vi "plcHMI_rev3.vi"() -> ()   [LabVIEW 2020]
doc: "ADS continuos synchronous write example using base blocks. \n\nThe client writes data synchronously and does wait for the respose from server."
uses:
  Agilent/AgilentTotalCluster.ctl
  Agilent/AgilentControl.ctl
  Agilent/Channel Config.ctl
  <vilib>/Platform/TimedLoop/XDataNode/timing_clust.ctl
  <vilib>/Platform/TimedLoop/XDataNode/nitl_modes.ctl
  <vilib>/Platform/TimedLoop/XDataNode/wakeup.ctl
  <userlib>/Beckhoff-LabVIEW-Interface/_DependsOn/With TypeResolving/Write Sync Single TypeResolved.vi
  <userlib>/Beckhoff-LabVIEW-Interface/_DependsOn/With TypeResolving/Read Sync Single TypeResolved.vi
  <vilib>/Platform/TimedLoop/XDataNode/XDataNode.xnode
  <vilib>/Platform/TimedLoop/XDataNode/XDNodeRunTimeDep.lvlib
panel:
  in  "Tab Control":T1(tab)
  out "error out":errorcluster
  in  "Symbol file path - MUST BE ENTERED\nLoad \"ADS Write AND Read Symbols REV X.X.xml\"":path
  out "bHasMached":bool
  out "Write Status":bool
  out "Read Status":bool
  in  "EXIT HMI":bool caption="STOP HMI\nEXIT HMI"
  out "Internal TwinCAT Handle ID Maps":dbl format="%#_12g"
  in  "802L TDK PSU Voltage Rating (abs(Volts))":i32=12000 min=1 max=50000
  in  "802L TDL PSU Peak Power (J/s)":i32=9000 min=1 max=50000
  in  "HVPS Model":u16(ring) items=["802L-12kV,9000J/s", "802L+50kV,9000J/s", "Other"]
  out "Test Interval Fault":bool
  in  "Cycle Time (Sec)":i32=15 min=0
  in  "Voltage Held by PSU":bool
  in  "Log Capacitor Voltage":bool
  in  "Log Temperature Data":bool
  out "Time Since Last Shot":string caption="Elapsed Time Text"
  in  "Duty Cycle":dbl
  in  "Current Control":bool
  out "Expected Voltage":i16
  in  "Dump":bool
  out "EOC":bool
  out "Maximum Test Number Reached":bool
  out "SCR Ready":bool
  in  "START":bool
  in  "STOP":bool
  in  "Hold":bool
  in  "Charge":bool
  in  "Shot":bool
  in  "HV Switch Mode":bool
  in  "CLEAR FAULT":bool
  in  "Manual/Auto":bool=TRUE
  out "Test Interval (Sec)":i32=15 min=0
  in  "Capacitance (uF)":sgl=1e-13 min=0 max=10000 format="%#_6f"
  in  "Target Charge Volt (V) - Min 1500V - TEMPORARY LIMIT 12kV":i32 min=-12000 max=12000 step=1
  out "Estimated Charge Time (seconds)":sgl
  in  "Hold Time Before Shot (seconds)":sgl max=1000
  in  "Max Number of Shots (Test intervals)":i16=1 min=1
  out "Shot Number":i16
  out "Charge Fault":bool=TRUE
  out "Discharge Fault":bool=TRUE
  out "Hold Fault":bool=TRUE
  out "Cap 1 Temp\nExceeded Fault":bool=TRUE
  out "Ambient Temp\nExceeded Fault":bool=TRUE
  out "PSU Fault":bool=TRUE
  out "Control Sys Fault":bool=TRUE
  out "test Running":bool
  out "Test State":string
  out "Cap 1 Voltage":i16
  out "Cap 1 Temperature":i16
  in  "Capacitor Voltage Data Log File Path (.xlsx)":path
  out "Load Temperature":i16
  out "Soft Dump Temp":i16
  out "Ambient Temp":i16
  out "Waveform Chart - Capacitor Voltage (Probe, abs(Volts))":dbl(graph)
  in  "Manual Charge Time (seconds)":sgl max=90
  in  "Reset Test Number":bool
  in  "Cap 1 Fault Temp (Cel)":i16 min=0 max=125
  in  "Capacitor Temperature Data Log File Path (.xlsx)":path
  out "Cap 1 Voltage (HVPS)":i16
  out "Capacitor Voltage":cluster{dbl, dbl}(graph)
  out "EOC":i16(graph)
  out "Soft Exception":bool
  out "PSU HV FB Fault":bool
  out "Charge FB Fault":bool
  out "Softdump FB Fault":bool
  out "SCR FB":i16(graph)
  in  "CH4 Vertical Units":string(combo)="V"
  in  "CH4 Vertical Units/div":dbl=2.0
  in  "Toggle Scope Scale":bool
  in  "CH1 Vertical Units/div":dbl=2.0
  in  "CH1 Vertical Units":string(combo)="V"
  in  "Horizontal Units":enum16{"us", "ms", "s"}(ring)
  in  "Horizontal Units/div":dbl=200.0
  out "Download":bool
  in  "Single":bool
  in  "Stop":bool
  out "Scope Trig":bool
  in  "Agilent Array":T2[](array[typedef])
  out "Process Step":u8
  in  "C:\\HVTest\\Local_Cap_Log_Scope (.xlsx)":path
  out "Stop Loops":bool
  # "CONFIGURATION"
  # "Press STOP HMI instead of\nLabView Abort Execution"
  # "PSU V Rating, Peak Power\nactive when OTHER\nis selected"
  # "INPUT VARIABLES - For TDK Lambda 802L\nMust be written to before START"
  # "FAULT STATUSES"
  # "Set to -1 for automated\nfull charge to setpoint"
  # "MANUAL CONTROLS"
  # "Does not record during \"wait\" and appends to data file. Must be named with .xlsx"
  # "HV Switch Configuration"
  # "Records during \"Test Running.\" Must be named with .xlsx"
  # "Control Sys Faults"
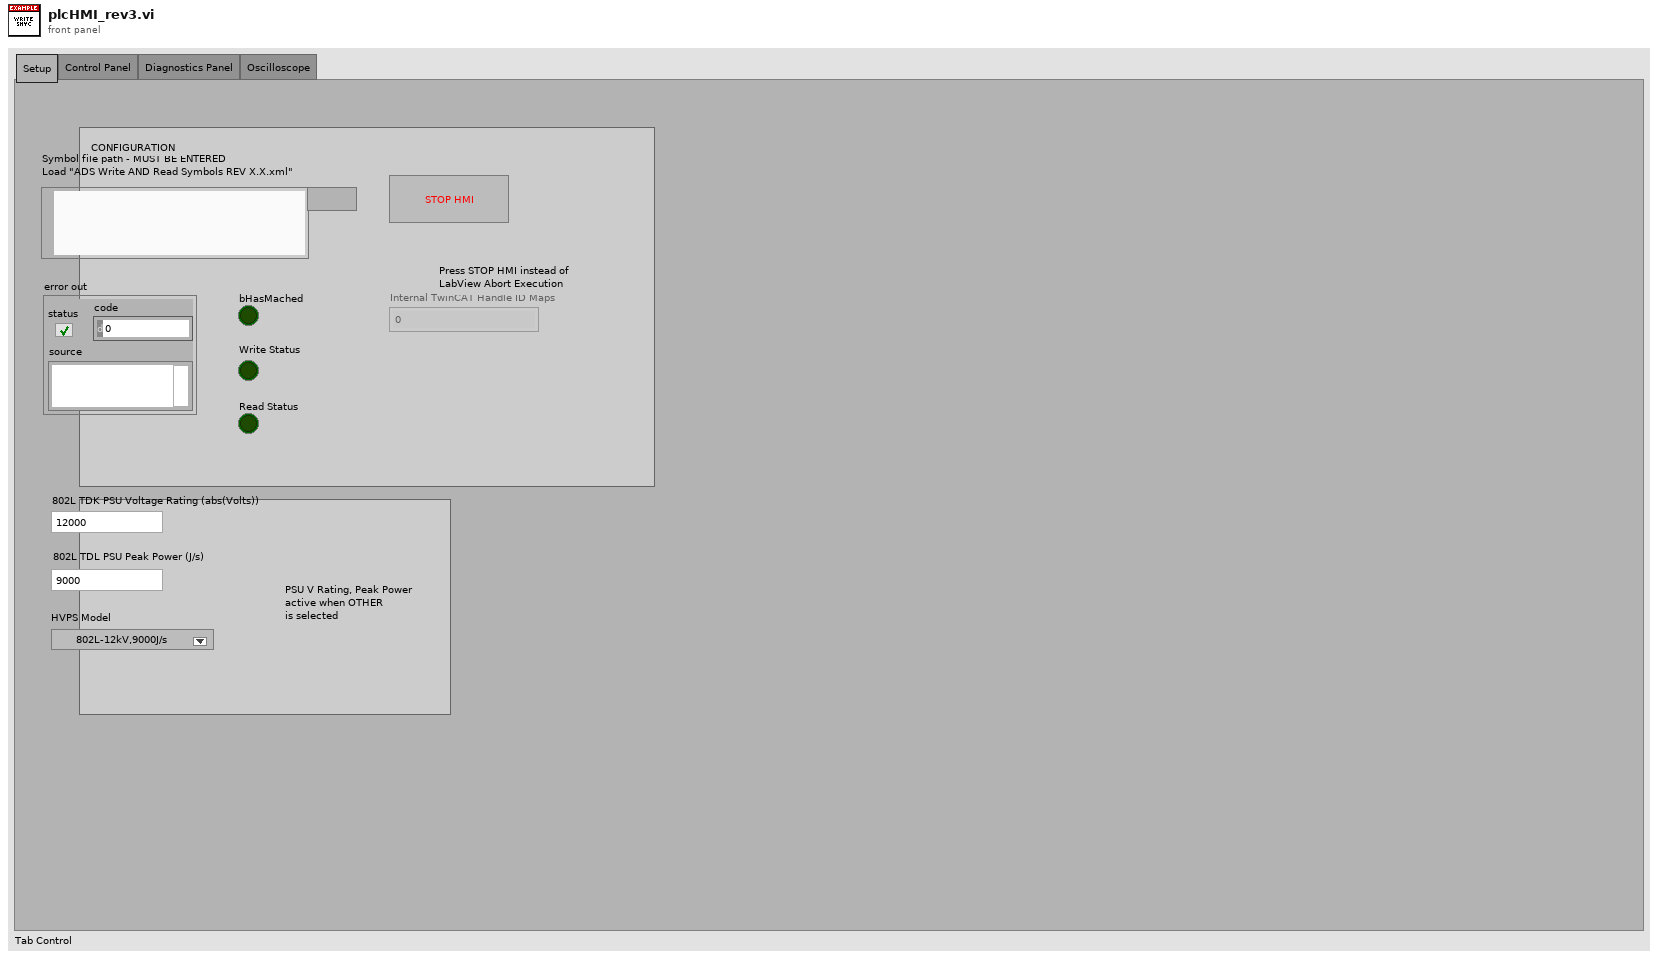
[diagram p1: front panel]
types:
  T1 = enum32{"Setup", "Control Panel", "Diagnostics Panel", "Oscilloscope"}
  T2 = typedef "AgilentTotalCluster.ctl" = cluster{"Agilent Graph":waveform(dbl)[], "Agilent Control":T3, "Agilent Setup Error":errorcluster, "Agilent Present":bool, "Enabled":bool}
  T3 = typedef "AgilentControl.ctl" = cluster{"Trig?":bool, "VISA session":refnum<visa-resource-name>, "Setup to Load":string, "Timeout (ms)":u32, "Desired Samp":enum32{"100", "250", "500", "1000", "2000", "5000", "10000", "20000", "50000", "100000", "200000", "500000", "1000000", "2000000", "4000000", "8000000"}, "Captured Samp":i32, "Desired Channels":T4[]}
  T4 = typedef "Channel Config.ctl" = cluster{"Chan Index":enum16{"Channel1", "Channel2", "Channel3", "Channel4", "MATH"}, "Name":string, "Samples":i32}
  T5 = typedef "XDNodeRunTimeDep.lvlib/timing_clust.ctl" = cluster{"Expected End [f-1]":u64, "Actual End [f-1]":u64, "Finished Late? [f-1]":bool, "Expected End [i-1]":u64, "Actual End [i-1]":u64, "Finished Late? [i-1]":bool, "Expected Start [i]":u64, "Actual Start [i]":u64, "Expected Start [f]":u64, "Actual Start [f]":u64, "Source Name":string, "Structure Name":string, "Period":i64, "Deadline":i64, "Offset":i64, "Start":i64, "Priority":i32, "Timeout":i32, "Mode":T6, "Wakeup Reason":T7, "Error":errorcluster, "Source Type":string, "Secondary Source Type":string, "Global End Time":u64, "Global Start Time":u64, "Frame Duration":u64, "Iteration Duration":u64, "Assigned CPU":i32, "I/O Scan Engine Mode":u32}
  T6 = typedef "XDNodeRunTimeDep.lvlib/nitl_modes.ctl" = enum32{"No Change", "Process missed periods, maintain original phase", "Discard missed periods, maintain original phase", "Process missed periods, ignore original phase", "Discard missed periods, ignore original phase"}
  T7 = typedef "XDNodeRunTimeDep.lvlib/wakeup.ctl" = enum32{"Normal", "Aborted", "Asynchronous wakeup", "Timing source error", "Timed loop error", "Timeout"}
  T8 = cluster{"Agilent Array[0]":T2, "Agilent Array[1]":T2, "Agilent Array[2]":T2, "Agilent Array[3]":T2, "Agilent Array[4]":T2, "Agilent Array[5]":T2, "Agilent Array[6]":T2, "Agilent Array[7]":T2, "Agilent Array[8]":T2}
  T9 = enum32{"100", "250", "500", "1000", "2000", "5000", "10000", "20000", "50000", "100000", "200000", "500000", "1000000", "2000000", "4000000", "8000000"}
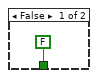
[diagram p2: hidden frame]
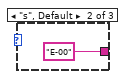
[diagram p5: hidden frame]
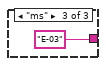
[diagram p6: hidden frame]
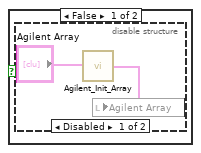
[diagram p7: hidden frame]
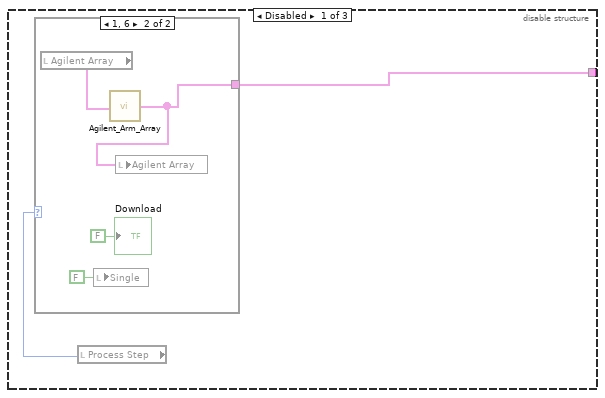
[diagram p11: hidden frame]
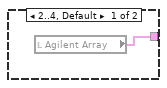
[diagram p12: hidden frame]
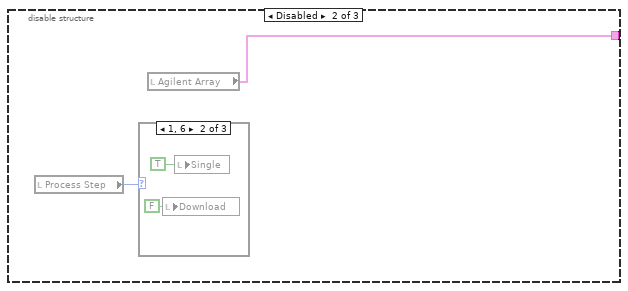
[diagram p13: hidden frame]
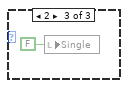
[diagram p15: hidden frame]
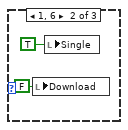
[diagram p17: hidden frame]
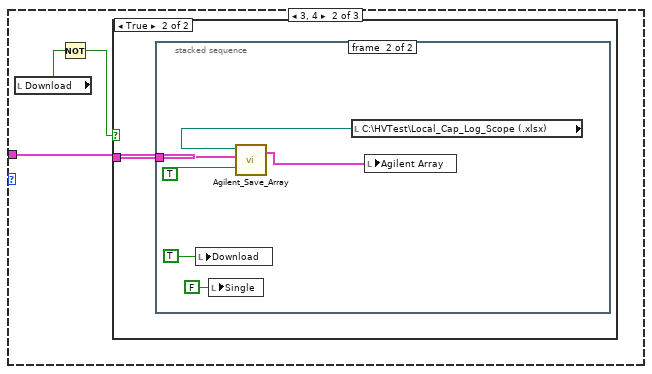
[diagram p19: hidden frame]
diagram:
  w105 = u16 17 items=["SyncLatest"=17, "AsyncLatest"=33] ("WriterMode")
  w189 = u16 33 items=["SyncLatest"=17, "AsyncLatest"=33] ("WriterMode")
  w228 = u16 33 items=["SyncLatest"=17, "AsyncLatest"=33] ("WriterMode")
  w247 = u16 33 items=["SyncLatest"=17, "AsyncLatest"=33] ("WriterMode")
  w266 = u16 33 items=["SyncLatest"=17, "AsyncLatest"=33] ("WriterMode")
  w285 = u16 33 items=["SyncLatest"=17, "AsyncLatest"=33] ("WriterMode")
  w304 = u16 33 items=["SyncLatest"=17, "AsyncLatest"=33] ("WriterMode")
  w323 = u16 33 items=["SyncLatest"=17, "AsyncLatest"=33] ("WriterMode")
  w342 = u16 17 items=["SyncLatest"=17, "AsyncLatest"=33] ("WriterMode")
  w361 = u16 17 items=["SyncLatest"=17, "AsyncLatest"=33] ("WriterMode")
  w380 = u16 17 items=["SyncLatest"=17, "AsyncLatest"=33] ("WriterMode")
  w399 = u16 17 items=["SyncLatest"=17, "AsyncLatest"=33] ("WriterMode")
  w418 = u16 17 items=["SyncLatest"=17, "AsyncLatest"=33] ("WriterMode")
  w437 = u16 17 items=["SyncLatest"=17, "AsyncLatest"=33] ("WriterMode")
  w456 = u16 17 items=["SyncLatest"=17, "AsyncLatest"=33] ("WriterMode")
  w471 = u16 17 items=["SyncLatest"=17, "AsyncLatest"=33] ("WriterMode")
  # "Variables/ Control"
  # "Documentation:\nCode separated vertically into two main sections - Write and read\nThey are further separated into BOOL and numeric\nThe OR gates wire all the error lines and the EXIT HMI button to a WHILE LOOP STOP\nThere current delay time on the routine is 100ms\nAll the AND gates connect the typecast resolve lines to the bHasMatched indicator\nThe second and third set of AND gates connect the write statuses to the Write Status indicator\nThe same is done for the read status indicator"
  # "WRITE NUMERICS"
  # "WRITE BOOLS"
  # "Select Symbol N"
  # "Read Initialization"
  # "Release \nTypeResolver"
  # "Release Writer"
  # "Send Request"
  # "Init \nTypeResolver"
  # "Init Writer"
  # "Select Symbol"
  # "Initialization"
  # "Call Release handle block\nat the end, when all nodes\nhave finished their execution"
  # "There must be only one release\nafter every init block.\nRelease block must be called\nalways at the end."
  # "Release"
  # "Symbol Interface"
  n1 = disable-structure shown="Enabled" {
    disable-tunnel: [w477 _] -> w475
    disable-tunnel: [w476 w479] -> w474
    frame Disabled {
      # "Using Symbol Interface"
      n2 = call <userlib>:"Symbol Interface.vi"() -> ("PortInfo"=w476:string, "error out"=w477:errorcluster)  [unwired: 14 in]
    }
    frame Enabled {
      # "Using Symbol File"
      n3 = Path To String(path="Symbol file path - MUST BE ENTERED\nLoad \"ADS Write AND Read Symbols REV X.X.xml\"") -> (string=w479:string)
    }
  }
  n4 = call <userlib>:"Init.vi"("XMLDescription"=w474, "error in (no error)"=w475) -> ("Handle"=w43:u32, "ReadGrpSymbols"=w25:string[], "WriteGrpSymbols"=w31:string[], "error out"=w11:errorcluster)  [unwired: 9 in, 1 out]
  n5 = Index Array(array=w31, index=0) -> (element=w10:string)
  n6 = Index Array(array=w31, index=21) -> (element=w30:string)
  n7 = Index Array(array=w31, index=20) -> (element=w36:string)
  n8 = Index Array(array=w31, index=14) -> (element=w229:string)
  n9 = Index Array(array=w31, index=9) -> (element=w324:string)
  n10 = Index Array(array=w31, index=10) -> (element=w305:string)
  n11 = Index Array(array=w31, index=12) -> (element=w267:string)
  n12 = Index Array(array=w31, index=11) -> (element=w286:string)
  n13 = Index Array(array=w31, index=13) -> (element=w248:string)
  n14 = Index Array(array=w31, index=18) -> (element=w44:string)
  n15 = Index Array(array=w31, index=19) -> (element=w37:string)
  n16 = Index Array(array=w31, index=7) -> (element=w343:string)
  n17 = Index Array(array=w31, index=2) -> (element=w438:string)
  n18 = Index Array(array=w31, index=3) -> (element=w419:string)
  n19 = Index Array(array=w31, index=5) -> (element=w381:string)
  n20 = Index Array(array=w31, index=4) -> (element=w400:string)
  n21 = Index Array(array=w31, index=6) -> (element=w362:string)
  n22 = Index Array(array=w31, index=1) -> (element=w457:string)
  n23 = Index Array(array=w31, index=16) -> (element=w126:string)
  n24 = Index Array(array=w31, index=8) -> (element=w104:string)
  n25 = Index Array(array=w31, index=15) -> (element=w190:string)
  n26 = Index Array(array=w31, index=17) -> (element=w90:string)
  n27 = call <userlib>:"Init Writer.vi"("Handle"=w43, "SymbolName"=w229, "WriterMode"=w228, "error constant"=w11) -> ("Handle"=w227:u32, "SymbolName"=w226:string, "WriterMode"=w225:u16, "WriteHandle"=w224:u32, "error IO"=w223:errorcluster)  [unwired: 7 in]
  n28 = call <userlib>:"Init Writer.vi"("Handle"=w43, "SymbolName"=w324, "WriterMode"=w323, "error constant"=w11) -> ("Handle"=w319:u32, "SymbolName"=w318:string, "WriterMode"=w317:u16, "WriteHandle"=w315:u32, "error IO"=w316:errorcluster)  [unwired: 7 in]
  n29 = call <userlib>:"Init Writer.vi"("Handle"=w43, "SymbolName"=w305, "WriterMode"=w304, "error constant"=w11) -> ("Handle"=w303:u32, "SymbolName"=w302:string, "WriterMode"=w301:u16, "WriteHandle"=w300:u32, "error IO"=w299:errorcluster)  [unwired: 7 in]
  n30 = call <userlib>:"Init Writer.vi"("Handle"=w43, "SymbolName"=w267, "WriterMode"=w266, "error constant"=w11) -> ("Handle"=w265:u32, "SymbolName"=w264:string, "WriterMode"=w263:u16, "WriteHandle"=w262:u32, "error IO"=w261:errorcluster)  [unwired: 7 in]
  n31 = call <userlib>:"Init Type.vi"("Handle"=w43, "SymbolName"=w229, "error in"=w11) -> ("Handle"=w222:u32, "TypeHdl"=w221:u32, "error IO"=w220:errorcluster)  [unwired: 7 in, 3 out]
  n32 = call <userlib>:"Init Type.vi"("Handle"=w43, "SymbolName"=w324, "error in"=w11) -> ("Handle"=w308:u32, "TypeHdl"=w307:u32, "error IO"=w306:errorcluster)  [unwired: 7 in, 3 out]
  n33 = call <userlib>:"Init Type.vi"("Handle"=w43, "SymbolName"=w305, "error in"=w11) -> ("Handle"=w298:u32, "TypeHdl"=w297:u32, "error IO"=w296:errorcluster)  [unwired: 7 in, 3 out]
  n34 = call <userlib>:"Init Writer.vi"("Handle"=w43, "SymbolName"=w286, "WriterMode"=w285, "error constant"=w11) -> ("Handle"=w284:u32, "SymbolName"=w283:string, "WriterMode"=w282:u16, "WriteHandle"=w281:u32, "error IO"=w280:errorcluster)  [unwired: 7 in]
  n35 = call <userlib>:"Init Type.vi"("Handle"=w43, "SymbolName"=w267, "error in"=w11) -> ("Handle"=w260:u32, "TypeHdl"=w259:u32, "error IO"=w258:errorcluster)  [unwired: 7 in, 3 out]
  n36 = call <userlib>:"Init Writer.vi"("Handle"=w43, "SymbolName"=w248, "WriterMode"=w247, "error constant"=w11) -> ("Handle"=w246:u32, "SymbolName"=w245:string, "WriterMode"=w244:u16, "WriteHandle"=w243:u32, "error IO"=w242:errorcluster)  [unwired: 7 in]
  n37 = call <userlib>:"Init Type.vi"("Handle"=w43, "SymbolName"=w286, "error in"=w11) -> ("Handle"=w279:u32, "TypeHdl"=w278:u32, "error IO"=w277:errorcluster)  [unwired: 7 in, 3 out]
  n38 = call <userlib>:"Init Type.vi"("Handle"=w43, "SymbolName"=w248, "error in"=w11) -> ("Handle"=w241:u32, "TypeHdl"=w240:u32, "error IO"=w239:errorcluster)  [unwired: 7 in, 3 out]
  n39 = call <userlib>:"Init Writer.vi"("Handle"=w43, "SymbolName"=w343, "WriterMode"=w342, "error constant"=w11) -> ("Handle"=w341:u32, "SymbolName"=w340:string, "WriterMode"=w339:u16, "WriteHandle"=w338:u32, "error IO"=w337:errorcluster)  [unwired: 7 in]
  n40 = call <userlib>:"Init Writer.vi"("Handle"=w43, "SymbolName"=w438, "WriterMode"=w437, "error constant"=w11) -> ("Handle"=w433:u32, "SymbolName"=w432:string, "WriterMode"=w431:u16, "WriteHandle"=w429:u32, "error IO"=w430:errorcluster)  [unwired: 7 in]
  n41 = call <userlib>:"Init Writer.vi"("Handle"=w43, "SymbolName"=w419, "WriterMode"=w418, "error constant"=w11) -> ("Handle"=w417:u32, "SymbolName"=w416:string, "WriterMode"=w415:u16, "WriteHandle"=w414:u32, "error IO"=w413:errorcluster)  [unwired: 7 in]
  n42 = call <userlib>:"Init Writer.vi"("Handle"=w43, "SymbolName"=w381, "WriterMode"=w380, "error constant"=w11) -> ("Handle"=w379:u32, "SymbolName"=w378:string, "WriterMode"=w377:u16, "WriteHandle"=w376:u32, "error IO"=w375:errorcluster)  [unwired: 7 in]
  n43 = call <userlib>:"Init Type.vi"("Handle"=w43, "SymbolName"=w343, "error in"=w11) -> ("Handle"=w336:u32, "TypeHdl"=w335:u32, "error IO"=w334:errorcluster)  [unwired: 7 in, 3 out]
  n44 = call <userlib>:"Init Type.vi"("Handle"=w43, "SymbolName"=w438, "error in"=w11) -> ("Handle"=w422:u32, "TypeHdl"=w421:u32, "error IO"=w420:errorcluster)  [unwired: 7 in, 3 out]
  n45 = call <userlib>:"Init Type.vi"("Handle"=w43, "SymbolName"=w419, "error in"=w11) -> ("Handle"=w412:u32, "TypeHdl"=w411:u32, "error IO"=w410:errorcluster)  [unwired: 7 in, 3 out]
  n46 = call <userlib>:"Init Writer.vi"("Handle"=w43, "SymbolName"=w400, "WriterMode"=w399, "error constant"=w11) -> ("Handle"=w398:u32, "SymbolName"=w397:string, "WriterMode"=w396:u16, "WriteHandle"=w395:u32, "error IO"=w394:errorcluster)  [unwired: 7 in]
  n47 = call <userlib>:"Init Type.vi"("Handle"=w43, "SymbolName"=w381, "error in"=w11) -> ("Handle"=w374:u32, "TypeHdl"=w373:u32, "error IO"=w372:errorcluster)  [unwired: 7 in, 3 out]
  n48 = call <userlib>:"Init Writer.vi"("Handle"=w43, "SymbolName"=w362, "WriterMode"=w361, "error constant"=w11) -> ("Handle"=w360:u32, "SymbolName"=w359:string, "WriterMode"=w358:u16, "WriteHandle"=w357:u32, "error IO"=w356:errorcluster)  [unwired: 7 in]
  n49 = call <userlib>:"Init Type.vi"("Handle"=w43, "SymbolName"=w400, "error in"=w11) -> ("Handle"=w393:u32, "TypeHdl"=w392:u32, "error IO"=w391:errorcluster)  [unwired: 7 in, 3 out]
  n50 = call <userlib>:"Init Type.vi"("Handle"=w43, "SymbolName"=w362, "error in"=w11) -> ("Handle"=w355:u32, "TypeHdl"=w354:u32, "error IO"=w353:errorcluster)  [unwired: 7 in, 3 out]
  n51 = call <userlib>:"Init Writer.vi"("Handle"=w43, "SymbolName"=w457, "WriterMode"=w456, "error constant"=w11) -> ("Handle"=w455:u32, "SymbolName"=w454:string, "WriterMode"=w453:u16, "WriteHandle"=w452:u32, "error IO"=w451:errorcluster)  [unwired: 7 in]
  n52 = call <userlib>:"Init Writer.vi"("Handle"=w43, "SymbolName"=w126, "error constant"=w11) -> ("Handle"=w125:u32, "SymbolName"=w124:string, "WriterMode"=w123:u16, "WriteHandle"=w121:u32, "error IO"=w122:errorcluster)  [unwired: 8 in]
  n53 = call <userlib>:"Init Type.vi"("Handle"=w43, "SymbolName"=w457, "error in"=w11) -> ("Handle"=w450:u32, "TypeHdl"=w449:u32, "error IO"=w448:errorcluster)  [unwired: 7 in, 3 out]
  n54 = call <userlib>:"Init Type.vi"("Handle"=w43, "SymbolName"=w126, "error in"=w11) -> ("Handle"=w120:u32, "TypeHdl"=w119:u32, "error IO"=w118:errorcluster)  [unwired: 7 in, 3 out]
  n55 = call <userlib>:"Init Writer.vi"("Handle"=w43, "SymbolName"=w10, "WriterMode"=w471, "error constant"=w11) -> ("Handle"=w470:u32, "SymbolName"=w469:string, "WriterMode"=w468:u16, "WriteHandle"=w467:u32, "error IO"=w466:errorcluster)  [unwired: 7 in]
  n56 = call <userlib>:"Init Type.vi"("Handle"=w43, "SymbolName"=w10, "error in"=w11) -> ("Handle"=w465:u32, "TypeHdl"=w464:u32, "error IO"=w459:errorcluster)  [unwired: 7 in, 3 out]
  n57 = call <userlib>:"Init Writer.vi"("Handle"=w43, "SymbolName"=w190, "WriterMode"=w189, "error constant"=w11) -> ("Handle"=w185:u32, "SymbolName"=w184:string, "WriterMode"=w183:u16, "WriteHandle"=w175:u32, "error IO"=w182:errorcluster)  [unwired: 7 in]
  n58 = call <userlib>:"Init Type.vi"("Handle"=w43, "SymbolName"=w190, "error in"=w11) -> ("Handle"=w180:u32, "TypeHdl"=w178:u32, "error IO"=w179:errorcluster)  [unwired: 7 in, 3 out]
  n59 = call <userlib>:"Init Writer.vi"("Handle"=w43, "SymbolName"=w90, "error constant"=w11) -> ("Handle"=w87:u32, "SymbolName"=w86:string, "WriterMode"=w85:u16, "WriteHandle"=w84:u32, "error IO"=w83:errorcluster)  [unwired: 8 in]
  n60 = call <userlib>:"Init Type.vi"("Handle"=w43, "SymbolName"=w90, "error in"=w11) -> ("Handle"=w82:u32, "TypeHdl"=w81:u32, "error IO"=w80:errorcluster)  [unwired: 7 in, 3 out]
  n61 = Index Array(array=w25, index=2) -> (element=w171:string)
  n62 = Index Array(array=w25, index=4) -> (element=w167:string)
  n63 = call <userlib>:"Init Writer.vi"("Handle"=w43, "SymbolName"=w104, "WriterMode"=w105, "error constant"=w11) -> ("Handle"=w103:u32, "SymbolName"=w102:string, "WriterMode"=w101:u16, "WriteHandle"=w100:u32, "error IO"=w99:errorcluster)  [unwired: 7 in]
  n64 = Index Array(array=w25, index=1) -> (element=w207:string)
  n65 = Index Array(array=w25, index=21) -> (element=w58:string)
  n66 = Index Array(array=w25, index=22) -> (element=w55:string)
  n67 = call <userlib>:"Init Type.vi"("Handle"=w43, "SymbolName"=w104, "error in"=w11) -> ("Handle"=w98:u32, "TypeHdl"=w97:u32, "error IO"=w96:errorcluster)  [unwired: 7 in, 3 out]
  n68 = Index Array(array=w25, index=0) -> (element=w206:string)
  n69 = Index Array(array=w25, index=3) -> (element=w168:string)
  n70 = Index Array(array=w25, index=20) -> (element=w63:string)
  n71 = Index Array(array=w25, index=23) -> (element=w54:string)
  n72 = Index Array(array=w25, index=16) -> (element=w173:string)
  n73 = Index Array(array=w25, index=24) -> (element=w52:string)
  n74 = Index Array(array=w25, index=11) -> (element=w195:string)
  n75 = Index Array(array=w25, index=10) -> (element=w196:string)
  n76 = Index Array(array=w25, index=17) -> (element=w66:string)
  n77 = Index Array(array=w25, index=18) -> (element=w65:string)
  n78 = Index Array(array=w25, index=13) -> (element=w193:string)
  n79 = Index Array(array=w25, index=27) -> (element=w23:string)
  n80 = Index Array(array=w25, index=12) -> (element=w194:string)
  n81 = Index Array(array=w25, index=15) -> (element=w191:string)
  n82 = Index Array(array=w25, index=19) -> (element=w64:string)
  n83 = Index Array(array=w25, index=26) -> (element=w24:string)
  n84 = Index Array(array=w25, index=5) -> (element=w77:string)
  n85 = Index Array(array=w25, index=6) -> (element=w161:string)
  n86 = Index Array(array=w25, index=9) -> (element=w205:string)
  n87 = Index Array(array=w25, index=14) -> (element=w192:string)
  n88 = Index Array(array=w25, index=8) -> (element=w163:string)
  n89 = Index Array(array=w25, index=25) -> (element=w41:string)
  n90 = Index Array(array=w25, index=7) -> (element=w162:string)
  n91 = node-c288(i64 10 ("Period")) -> (w113:T5)  [unwired: 2 in]
  n92 = timed-loop {
    tunnel: w470 -> [w791]
    tunnel: w469 -> [w790]
    tunnel: w468 -> [w789]
    tunnel: w467 -> [w788]
    tunnel: w465 -> [w1060]
    tunnel: w464 -> [w1059]
    tunnel: [w786] -> w463
    tunnel: [w785] -> w462
    tunnel: [w1058] -> w461
    tunnel: [w1057] -> w460
    tunnel: w455 -> [w1055]
    tunnel: w454 -> [w1054]
    tunnel: w453 -> [w1053]
    tunnel: w452 -> [w1052]
    tunnel: w450 -> [w1050]
    tunnel: w449 -> [w1049]
    tunnel: [w1047] -> w446
    tunnel: [w1046] -> w445
    tunnel: [w1045] -> w443
    tunnel: [w1044] -> w442
    tunnel: w433 -> [w1043]
    tunnel: w432 -> [w1042]
    tunnel: w431 -> [w1041]
    tunnel: w429 -> [w1039]
    tunnel: [w1038] -> w428
    tunnel: [w1037] -> w427
    tunnel: [w1036] -> w424
    tunnel: [w1035] -> w423
    tunnel: w422 -> [w1034]
    tunnel: w421 -> [w1033]
    tunnel: w417 -> [w1031]
    tunnel: w416 -> [w1030]
    tunnel: w415 -> [w1029]
    tunnel: w414 -> [w1028]
    tunnel: w412 -> [w1026]
    tunnel: w411 -> [w1025]
    tunnel: [w1023] -> w408
    tunnel: [w1022] -> w407
    tunnel: [w1021] -> w405
    tunnel: [w1020] -> w404
    tunnel: w398 -> [w1019]
    tunnel: w397 -> [w1018]
    tunnel: w396 -> [w1017]
    tunnel: w395 -> [w1016]
    tunnel: w393 -> [w1014]
    tunnel: w392 -> [w1013]
    tunnel: [w1011] -> w389
    tunnel: [w1010] -> w388
    tunnel: [w1009] -> w386
    tunnel: [w1008] -> w385
    tunnel: w379 -> [w1007]
    tunnel: w378 -> [w1006]
    tunnel: w377 -> [w1005]
    tunnel: w376 -> [w1004]
    tunnel: w374 -> [w1002]
    tunnel: w373 -> [w1001]
    tunnel: [w999] -> w370
    tunnel: [w998] -> w369
    tunnel: [w997] -> w367
    tunnel: [w996] -> w366
    tunnel: w360 -> [w995]
    tunnel: w359 -> [w994]
    tunnel: w358 -> [w993]
    tunnel: w357 -> [w992]
    tunnel: w355 -> [w990]
    tunnel: w354 -> [w989]
    tunnel: [w987] -> w351
    tunnel: [w986] -> w350
    tunnel: [w985] -> w348
    tunnel: [w984] -> w347
    tunnel: w341 -> [w983]
    tunnel: w340 -> [w982]
    tunnel: w339 -> [w981]
    tunnel: w338 -> [w980]
    tunnel: w336 -> [w978]
    tunnel: w335 -> [w977]
    tunnel: [w975] -> w332
    tunnel: [w974] -> w331
    tunnel: [w973] -> w329
    tunnel: [w972] -> w328
    tunnel: w319 -> [w971]
    tunnel: w318 -> [w970]
    tunnel: w317 -> [w969]
    tunnel: w315 -> [w967]
    tunnel: [w966] -> w314
    tunnel: [w965] -> w313
    tunnel: [w964] -> w310
    tunnel: [w963] -> w309
    tunnel: w308 -> [w962]
    tunnel: w307 -> [w961]
    tunnel: w303 -> [w959]
    tunnel: w302 -> [w958]
    tunnel: w301 -> [w957]
    tunnel: w300 -> [w956]
    tunnel: w298 -> [w954]
    tunnel: w297 -> [w953]
    tunnel: [w951] -> w294
    tunnel: [w950] -> w293
    tunnel: [w949] -> w291
    tunnel: [w948] -> w290
    tunnel: w284 -> [w947]
    tunnel: w283 -> [w946]
    tunnel: w282 -> [w945]
    tunnel: w281 -> [w944]
    tunnel: w279 -> [w942]
    tunnel: w278 -> [w941]
    tunnel: [w939] -> w275
    tunnel: [w938] -> w274
    tunnel: [w937] -> w272
    tunnel: [w936] -> w271
    tunnel: w265 -> [w935]
    tunnel: w264 -> [w934]
    tunnel: w263 -> [w933]
    tunnel: w262 -> [w932]
    tunnel: w260 -> [w930]
    tunnel: w259 -> [w929]
    tunnel: [w927] -> w256
    tunnel: [w926] -> w255
    tunnel: [w925] -> w253
    tunnel: [w924] -> w252
    tunnel: w246 -> [w923]
    tunnel: w245 -> [w922]
    tunnel: w244 -> [w921]
    tunnel: w243 -> [w920]
    tunnel: w241 -> [w918]
    tunnel: w240 -> [w917]
    tunnel: [w915] -> w237
    tunnel: [w914] -> w236
    tunnel: [w913] -> w234
    tunnel: [w912] -> w233
    tunnel: w227 -> [w911]
    tunnel: w226 -> [w910]
    tunnel: w225 -> [w909]
    tunnel: w224 -> [w908]
    tunnel: w222 -> [w906]
    tunnel: w221 -> [w905]
    tunnel: [w903] -> w218
    tunnel: [w902] -> w217
    tunnel: [w901] -> w215
    tunnel: [w900] -> w214
    tunnel: w207 -> [w899]
    tunnel: w206 -> [w898]
    tunnel: w205 -> [w897]
    tunnel: [w896] -> w156
    tunnel: w196 -> [w895]
    tunnel: w195 -> [w894]
    tunnel: w194 -> [w893]
    tunnel: w193 -> [w892]
    tunnel: w192 -> [w891]
    tunnel: w191 -> [w890]
    tunnel: [w889] -> w110
    tunnel: [w888] -> w155
    tunnel: [w887] -> w154
    tunnel: [w886] -> w153
    tunnel: [w885] -> w152
    tunnel: [w828] -> w151
    tunnel: [w826] -> w150
    shift-right: [w714] -> w473
    shift-left: w466 -> [w787]
    shift-right: [w713] -> w472
    shift-left: w459 -> [w1056]
    shift-right: [w711] -> w444
    shift-left: w451 -> [w1051]
    shift-right: [w710] -> w441
    shift-left: w448 -> [w1048]
    shift-right: [w708] -> w426
    shift-left: w430 -> [w1040]
    shift-right: [w707] -> w425
    shift-left: w420 -> [w1032]
    shift-right: [w705] -> w406
    shift-left: w413 -> [w1027]
    shift-right: [w704] -> w403
    shift-left: w410 -> [w1024]
    shift-right: [w702] -> w387
    shift-left: w394 -> [w1015]
    shift-right: [w701] -> w384
    shift-left: w391 -> [w1012]
    shift-right: [w699] -> w368
    shift-left: w375 -> [w1003]
    shift-right: [w698] -> w365
    shift-left: w372 -> [w1000]
    shift-right: [w696] -> w349
    shift-left: w356 -> [w991]
    shift-right: [w695] -> w346
    shift-left: w353 -> [w988]
    shift-right: [w693] -> w330
    shift-left: w337 -> [w979]
    shift-right: [w692] -> w327
    shift-left: w334 -> [w976]
    shift-right: [w691] -> w312
    shift-left: w316 -> [w968]
    shift-right: [w690] -> w311
    shift-left: w306 -> [w960]
    shift-right: [w688] -> w292
    shift-left: w299 -> [w955]
    shift-right: [w687] -> w289
    shift-left: w296 -> [w952]
    shift-right: [w685] -> w273
    shift-left: w280 -> [w943]
    shift-right: [w684] -> w270
    shift-left: w277 -> [w940]
    shift-right: [w682] -> w254
    shift-left: w261 -> [w931]
    shift-right: [w681] -> w251
    shift-left: w258 -> [w928]
    shift-right: [w679] -> w235
    shift-left: w242 -> [w919]
    shift-right: [w678] -> w232
    shift-left: w239 -> [w916]
    shift-right: [w676] -> w216
    shift-left: w223 -> [w907]
    shift-right: [w675] -> w213
    shift-left: w220 -> [w904]
    tunnel: w185 -> [w868]
    tunnel: w184 -> [w867]
    tunnel: w183 -> [w866]
    tunnel: [w864] -> w9
    tunnel: [w863] -> w181
    tunnel: w180 -> [w862]
    tunnel: w178 -> [w860]
    tunnel: [w859] -> w177
    tunnel: [w858] -> w176
    tunnel: w175 -> [w857]
    tunnel: w173 -> [w856]
    tunnel: [w827] -> w149
    tunnel: [w850] -> w158
    tunnel: w11 -> [w849]
    tunnel: [w847] -> w157
    tunnel: w171 -> [w846]
    tunnel: w168 -> [w842]
    tunnel: w167 -> [w841]
    tunnel: [w832] -> w159
    tunnel: [w831] -> w160
    tunnel: w163 -> [w825]
    tunnel: w162 -> [w824]
    tunnel: w161 -> [w823]
    tunnel: [w810] -> w74
    tunnel: [w809] -> w73
    tunnel: [w808] -> w72
    tunnel: w125 -> [w489]
    tunnel: w124 -> [w490]
    tunnel: w123 -> [w802]
    tunnel: w121 -> [w800]
    tunnel: w120 -> [w799]
    tunnel: w119 -> [w798]
    tunnel: [w796] -> w116
    tunnel: [w795] -> w115
    tunnel: [w794] -> w8
    tunnel: [w793] -> w7
    timing: w113 -> [_]
    timing-out: [_] -> w112
    tunnel: w43 -> [w784]
    tunnel: [w671] -> w76
    tunnel: w103 -> [w666]
    tunnel: w102 -> [w665]
    tunnel: w101 -> [w664]
    tunnel: w100 -> [w663]
    tunnel: w98 -> [w661]
    tunnel: w97 -> [w660]
    tunnel: [w657] -> w95
    tunnel: [w656] -> w94
    tunnel: [w655] -> w93
    tunnel: [w654] -> w92
    tunnel: w87 -> [w644]
    tunnel: w86 -> [w643]
    tunnel: w85 -> [w642]
    tunnel: w84 -> [w641]
    tunnel: w82 -> [w639]
    tunnel: w81 -> [w638]
    tunnel: [w635] -> w15
    tunnel: [w632] -> w14
    tunnel: [w634] -> w12
    tunnel: [w633] -> w13
    tunnel: [w627] -> w75
    tunnel: w77 -> [w623]
    tunnel: [w622] -> w71
    tunnel: w66 -> [w617]
    tunnel: w65 -> [w612]
    tunnel: w64 -> [w611]
    tunnel: w63 -> [w610]
    tunnel: [w607] -> w62
    tunnel: [w605] -> w61
    tunnel: [w600] -> w60
    tunnel: [w599] -> w47
    tunnel: w58 -> [w597]
    tunnel: w55 -> [w572]
    tunnel: w54 -> [w571]
    tunnel: w52 -> [w564]
    tunnel: [w560] -> w51
    tunnel: [w559] -> w50
    tunnel: [w558] -> w49
    tunnel: [w557] -> w48
    tunnel: w44 -> [w556]
    tunnel: w43 -> [w518]
    tunnel: w11 -> [w555]
    tunnel: [w550] -> w35
    tunnel: [w549] -> _
    tunnel: w41 -> [w545]
    tunnel: [w541] -> w40
    tunnel: w37 -> [w540]
    tunnel: w36 -> [w539]
    tunnel: w11 -> [w514]
    tunnel: [w534] -> w34
    tunnel: [w533] -> w33
    tunnel: w30 -> [w519]
    tunnel: [w513] -> w29
    tunnel: w24 -> [w500]
    tunnel: w23 -> [w499]
    tunnel: [w494] -> w22
    tunnel: [w493] -> w21
    shift-right: [w488] -> w20
    shift-left: w182 -> [w865]
    shift-right: [w487] -> w19
    shift-left: w179 -> [w861]
    tunnel: w80 -> [w637]
    tunnel: [w483] -> w16
    tunnel: w118 -> [w797]
    tunnel: w83 -> [w640]
    tunnel: [w484] -> w17
    tunnel: w122 -> [w801]
    tunnel: [w485] -> w6
    tunnel: [w486] -> w18
    shift-right: [w481] -> w2
    shift-left: w99 -> [w662]
    shift-right: [w480] -> w1
    shift-left: w96 -> [w659]
    stop <- w618 stop-if-true
    # "Stop Loop on Error (OR gates)"
    # "Error Stop Loop AND"
    # "Typecast Match AND"
    # "Write Status AND"
    # "READ BOOLS"
    # "READ NUMERICS"
    # "STOP HMI via error or EXIT button"
    # "Check Read status and\nthen convert Variant \nto LabVIEW type (AND gates)"
    # "Sync Read Single"
    n93 = node-c288() -> (w672:errorcluster)  [unwired: 1 in]
    n94 = disable-structure shown="Enabled" {
      frame Enabled {
        n95 = flat-sequence {
          tunnel: [w1200] -> w1144
          tunnel: w1144 -> [w1219]
          frame #0 {
            n96 = disable-structure shown="Enabled" {
              frame Enabled {
                n97 = feedback #1(TRUE) -> (w1146:bool)
                n98 = And(x=TRUE, y=w1146) -> (x .and. y?=w1149:bool)
                n99 = case shown="True" w1149 {
                  tunnel: [FALSE FALSE] -> w1147
                  frame False {
                  }
                  frame True {
                    n100 = local read "Agilent Array"() -> (w1152:T2[])
                    n101 = call "Agilent_Init_Array.vi"("Agilent Array In"=w1152) -> ("Agilent Array Out"=w1153:T2[])
                    n102 = call "Agilent_Arm_Array.vi"("Agilent Array In"=w1153) -> ("Agilent Array Out"=w1151:T2[])
                    n103 = local write "Agilent Array"(w1151) -> ()
                  }
                }
                n104 = feedback-in #1(w1147) -> ()
              }
              frame Disabled {
              }
            }
          }
          frame #1 {
            n105 = case shown="True" "Toggle Scope Scale" {
              frame False {
              }
              frame True {
                n106 = Number To Decimal String(number="CH4 Vertical Units/div") -> (decimal integer string=w1159:string)  [unwired: 1 in]
                n107 = Number To Decimal String(number="Horizontal Units/div") -> (decimal integer string=w1167:string)  [unwired: 1 in]
                n108 = Number To Decimal String(number="CH1 Vertical Units/div") -> (decimal integer string=w1165:string)  [unwired: 1 in]
                n109 = case shown="\"us\"" "Horizontal Units" {
                  tunnel: ["E-06" "E-00" "E-03"] -> w1176
                  frame "us" {
                  }
                  frame "s", Default {
                  }
                  frame "ms" {
                  }
                }
                n110 = Concatenate Strings(":CHAN4:SCAL " ("write buffer"), w1159, "CH4 Vertical Units") -> (w1158:string)
                n111 = Concatenate Strings(":CHAN1:SCAL " ("write buffer"), w1165, "CH1 Vertical Units") -> (w1172:string)
                n112 = Concatenate Strings(":TIM:SCAL " ("write buffer"), w1167, w1176) -> (w1175:string)
                n113 = VISA Open(VISA resource name=refnum<visa-resource-name> "HV_Test_Scope") -> (VISA resource name=w1170:refnum<visa-resource-name>, error out=w1171:errorcluster)  [unwired: 4 in]
                n114 = VISA Write(VISA resource name=w1170, write buffer=w1175, error in (no error)=w1171) -> (VISA resource name out=w1179:refnum<visa-resource-name>, error out=w1178:errorcluster)  [unwired: 1 out]
                n115 = VISA Write(VISA resource name=w1179, write buffer=w1172, error in (no error)=w1178) -> (VISA resource name out=w1164:refnum<visa-resource-name>, error out=w1162:errorcluster)  [unwired: 1 out]
                n116 = VISA Write(VISA resource name=w1164, write buffer=w1158, error in (no error)=w1162) -> (VISA resource name out=w1163:refnum<visa-resource-name>, error out=w1161:errorcluster)  [unwired: 1 out]
                n117 = VISA Close(VISA resource name=w1163, error in (no error)=w1161) -> ()  [unwired: 1 out]
              }
            }
          }
          frame #2 {
            n118 = disable-structure shown="Enabled" {
              frame Enabled {
                n119 = case shown="True" "Stop" {
                  frame False {
                    n120 = disable-structure shown="Disabled" {
                      frame Disabled {
                        n121 = call "Agilent_Init_Array.vi"("Agilent Array In"="Agilent Array") -> ("Agilent Array Out"=w1186:T2[])
                        n122 = local write "Agilent Array"(w1186) -> ()
                      }
                      frame Enabled {
                      }
                    }
                  }
                  frame True {
                    n123 = VISA Open(VISA resource name=refnum<visa-resource-name> "HV_Test_Scope") -> (VISA resource name=w1192:refnum<visa-resource-name>, error out=w1193:errorcluster)  [unwired: 4 in]
                    n124 = VISA Write(VISA resource name=w1192, write buffer=":STOP", error in (no error)=w1193) -> (VISA resource name out=w1190:refnum<visa-resource-name>, error out=w1191:errorcluster)  [unwired: 1 out]
                    n125 = VISA Close(VISA resource name=w1190, error in (no error)=w1191) -> ()  [unwired: 1 out]
                  }
                }
              }
              frame Disabled {
              }
            }
            n126 = case shown="True" "Single" {
              frame False {
              }
              frame True {
                n127 = VISA Open(VISA resource name=refnum<visa-resource-name> "HV_Test_Scope") -> (VISA resource name=w1198:refnum<visa-resource-name>, error out=w1199:errorcluster)  [unwired: 4 in]
                n128 = VISA Write(VISA resource name=w1198, write buffer=":SINGLE", error in (no error)=w1199) -> (VISA resource name out=w1196:refnum<visa-resource-name>, error out=w1197:errorcluster)  [unwired: 1 out]
                n129 = VISA Close(VISA resource name=w1196, error in (no error)=w1197) -> ()  [unwired: 1 out]
              }
            }
          }
          frame #3 {
            n130 = disable-structure shown="Enabled" {
              disable-tunnel: [w1202 w1209 w1214] -> w1200
              frame Disabled {
                n131 = local read "Process Step"() -> (w1201:u8)
                n132 = case shown="1, 6" w1201 {
                  tunnel: [w1203 w1207] -> w1202
                  frame 2..4, Default {
                    n133 = local read "Agilent Array"() -> (w1203:T2[])
                  }
                  frame 1, 6 {
                    n134 = local read "Agilent Array"() -> (w1204:T2[])
                    n135 = local write "Single"(FALSE ("Single")) -> ()
                    n136 = call "Agilent_Arm_Array.vi"("Agilent Array In"=w1204) -> ("Agilent Array Out"=w1207:T2[])
                    n137 = local write "Agilent Array"(w1207) -> ()
                    "Download" <- FALSE ("Downloading")
                  }
                }
              }
              frame Disabled {
                n138 = local read "Process Step"() -> (w1208:u8)
                n139 = case shown="1, 6" w1208 {
                  frame 0, Default {
                  }
                  frame 1, 6 {
                    n140 = local write "Download"(FALSE ("Download")) -> ()
                    n141 = local write "Single"(TRUE ("Single")) -> ()
                  }
                  frame 2 {
                    n142 = local write "Single"(FALSE ("Single")) -> ()
                  }
                }
                n143 = local read "Agilent Array"() -> (w1209:T2[])
              }
              frame Enabled {
                n144 = local read "Process Step"() -> (w1213:u8)
                n145 = case shown="2, 7" w1213 {
                  frame 0, Default {
                  }
                  frame 1, 6 {
                    n146 = local write "Download"(FALSE ("Download")) -> ()
                    n147 = local write "Single"(TRUE ("Single")) -> ()
                  }
                  frame 2, 7 {
                    n148 = local write "Single"(FALSE ("Single")) -> ()
                  }
                }
                n149 = local read "Agilent Array"() -> (w1214:T2[])
              }
            }
          }
          frame #4 {
            n150 = local read "Process Step"() -> (w1218:u8)
            n151 = case shown="0" w1218 {
              tunnel: w1219 -> [_ w1222 w1235]
              frame Default {
              }
              frame 3, 4 {
                n152 = local read "Download"() -> (w1221:bool)
                n153 = Not(x=w1221) -> (.not. x?=w1220:bool)
                n154 = case shown="True" w1220 {
                  tunnel: w1222 -> [_ w1223]
                  frame False {
                  }
                  frame True {
                    n155 = stacked-sequence {
                      tunnel: w1223 -> [_ w1233]
                      frame #0 {
                        n156 = local read "Agilent Array"() -> (w1227:T2[])
                        n157 = Array To Cluster(array=w1227) -> (cluster=w1226:T8)
                        n158 = Unbundle By Name(w1226) -> ("Agilent Array[0].Agilent Control.Desired Samp"=w1224:T9)
                        n159 = call "GF_SetRecordLengthProperly.vi"("Num Samples"=w1224, "VISA resource name"=refnum<visa-resource-name> "HV_Test_Scope") -> ()  [unwired: 1 in, 2 out]
                      }
                      frame #1 {
                        n160 = local write "Download"(TRUE ("Downloading")) -> ()
                        n161 = local write "Single"(FALSE ("Single")) -> ()
                        n162 = local read "C:\\HVTest\\Local_Cap_Log_Scope (.xlsx)"() -> (w1228:path)
                        n163 = call "Agilent_Save_Array.vi"("Agilent Download"=TRUE, "Agilent Array In"=w1233, "File Path"=w1228) -> ("Agilent Array Out"=w1231:T2[])  [unwired: 1 in, 1 out]
                        n164 = local write "Agilent Array"(w1231) -> ()
                      }
                    }
                  }
                }
              }
              frame 0 {
                n165 = local read "Maximum Test Number Reached"() -> (w1234:bool)
                n166 = case shown="True" w1234 {
                  tunnel: w1235 -> [_ w1238]
                  frame False {
                  }
                  frame True {
                    n167 = local read "Download"() -> (w1237:bool)
                    n168 = Not(x=w1237) -> (.not. x?=w1236:bool)
                    n169 = case shown="True" w1236 {
                      tunnel: w1238 -> [_ w1239]
                      frame False {
                      }
                      frame True {
                        n170 = stacked-sequence {
                          tunnel: w1239 -> [_ w1249]
                          frame #0 {
                            n171 = local read "Agilent Array"() -> (w1243:T2[])
                            n172 = Array To Cluster(array=w1243) -> (cluster=w1242:T8)
                            n173 = Unbundle By Name(w1242) -> ("Agilent Array[0].Agilent Control.Desired Samp"=w1240:T9)
                            n174 = call "GF_SetRecordLengthProperly.vi"("Num Samples"=w1240, "VISA resource name"=refnum<visa-resource-name> "HV_Test_Scope") -> ()  [unwired: 1 in, 2 out]
                          }
                          frame #1 {
                            n175 = local write "Download"(TRUE ("Downloading")) -> ()
                            n176 = local write "Single"(FALSE ("Single")) -> ()
                            n177 = call "Agilent_Save_Array.vi"("Agilent Download"=TRUE, "Agilent Array In"=w1249, "File Path"="C:\\HVTest\\Local_Cap_Log_Scope (.xlsx)") -> ("Agilent Array Out"=w1247:T2[])  [unwired: 1 in, 1 out]
                            n178 = local write "Agilent Array"(w1247) -> ()
                          }
                        }
                      }
                    }
                  }
                }
              }
            }
          }
        }
      }
      frame Disabled {
      }
    }
    n179 = case shown="0, Default" "HVPS Model" {
      tunnel: ["802L TDK PSU Voltage Rating (abs(Volts))" 12000 50000] -> w792
      tunnel: ["802L TDL PSU Peak Power (J/s)" 9000 9000] -> w829
      frame 2 {
      }
      frame 0, Default {
      }
      frame 1 {
      }
    }
    n180 = flat-sequence {
      tunnel: w799 -> [w1357]
      tunnel: w798 -> [w1358]
      tunnel: w797 -> [w1355]
      tunnel: [w1355] -> w806
      tunnel: [w1358] -> w805
      tunnel: [w1357] -> w804
      tunnel: [w1356] -> w803
      tunnel: w806 -> [w1367]
      tunnel: w805 -> [w1366]
      tunnel: w804 -> [w1365]
      tunnel: w803 -> [w1360]
      tunnel: [w1362] -> w485
      tunnel: [w1364] -> w794
      tunnel: [w1359] -> w793
      tunnel: [w1363] -> w491
      tunnel: [w1361] -> w631
      frame #0 {
        # "Write Data"
        n181 = To Single Precision Float(number="Manual Charge Time (seconds)") -> (single precision float=w1353:sgl)
        n182 = To Variant(anything=w1353) -> (Variant=w1356:variant)
      }
      frame #1 {
        # "Resolve To TC"
        n183 = call <userlib>:"Resolve To TC Type.vi"("Handle"=w1365, "TypHdl"=w1366, "WData"=w1360, "error in"=w1367) -> ("Handle"=w1359:u32, "TypHdl"=w1364:u32, "bHasMatched"=w1361:bool, "ADSWData"=w1363:variant, "error out"=w1362:errorcluster)  [unwired: 7 in]
      }
    }
    n184 = flat-sequence {
      tunnel: w639 -> [w1270]
      tunnel: w638 -> [w1271]
      tunnel: w637 -> [w1268]
      tunnel: [w1268] -> w648
      tunnel: [w1271] -> w647
      tunnel: [w1270] -> w646
      tunnel: [w1269] -> w645
      tunnel: [w1274] -> w483
      tunnel: [w1277] -> w633
      tunnel: [w1276] -> w634
      tunnel: [w1275] -> w636
      tunnel: w648 -> [w1280]
      tunnel: w647 -> [w1279]
      tunnel: w646 -> [w1278]
      tunnel: w645 -> [w1273]
      tunnel: [w1272] -> w552
      frame #0 {
        # "Write Data"
        n185 = To Word Integer(number="Cap 1 Fault Temp (Cel)") -> (16bit integer=w1266:i16)
        n186 = To Variant(anything=w1266) -> (Variant=w1269:variant)
      }
      frame #1 {
        # "Resolve To TC"
        n187 = call <userlib>:"Resolve To TC Type.vi"("Handle"=w1278, "TypHdl"=w1279, "WData"=w1273, "error in"=w1280) -> ("Handle"=w1276:u32, "TypHdl"=w1277:u32, "bHasMatched"=w1272:bool, "ADSWData"=w1275:variant, "error out"=w1274:errorcluster)  [unwired: 7 in]
      }
    }
    n188 = flat-sequence {
      tunnel: w906 -> [w1482]
      tunnel: w905 -> [w1483]
      tunnel: w904 -> [w1484]
      tunnel: [w1484] -> w1088
      tunnel: [w1483] -> w1087
      tunnel: [w1482] -> w1086
      tunnel: [w1481] -> w1085
      tunnel: [w1487] -> w675
      tunnel: [w1490] -> w900
      tunnel: [w1489] -> w901
      tunnel: [w1488] -> w873
      tunnel: w1088 -> [w1493]
      tunnel: w1087 -> [w1492]
      tunnel: w1086 -> [w1491]
      tunnel: w1085 -> [w1485]
      tunnel: [w1486] -> w739
      frame #0 {
        # "Write Data"
        n189 = To Word Integer(number="Max Number of Shots (Test intervals)") -> (16bit integer=w1480:i16)
        n190 = To Variant(anything=w1480) -> (Variant=w1481:variant)
      }
      frame #1 {
        # "Resolve To TC"
        n191 = call <userlib>:"Resolve To TC Type.vi"("Handle"=w1491, "TypHdl"=w1492, "WData"=w1485, "error in"=w1493) -> ("Handle"=w1489:u32, "TypHdl"=w1490:u32, "bHasMatched"=w1486:bool, "ADSWData"=w1488:variant, "error out"=w1487:errorcluster)  [unwired: 7 in]
      }
    }
    n192 = flat-sequence {
      tunnel: w862 -> [w1377]
      tunnel: w860 -> [w1378]
      tunnel: w861 -> [w1379]
      tunnel: [w1379] -> w872
      tunnel: [w1378] -> w871
      tunnel: [w1377] -> w870
      tunnel: [w1376] -> w869
      tunnel: w829 -> [w1375]
      tunnel: [w1382] -> w487
      tunnel: [w1385] -> w858
      tunnel: [w1384] -> w859
      tunnel: [w1383] -> w492
      tunnel: w872 -> [w1388]
      tunnel: w871 -> [w1387]
      tunnel: w870 -> [w1386]
      tunnel: w869 -> [w1381]
      tunnel: [w1380] -> w741
      frame #0 {
        # "Write Data"
        n193 = To Long Integer(number=w1375) -> (32bit integer=w1374:i32)
        n194 = To Variant(anything=w1374) -> (Variant=w1376:variant)
      }
      frame #1 {
        # "Resolve To TC"
        n195 = call <userlib>:"Resolve To TC Type.vi"("Handle"=w1386, "TypHdl"=w1387, "WData"=w1381, "error in"=w1388) -> ("Handle"=w1384:u32, "TypHdl"=w1385:u32, "bHasMatched"=w1380:bool, "ADSWData"=w1383:variant, "error out"=w1382:errorcluster)  [unwired: 7 in]
      }
    }
    n196 = flat-sequence {
      tunnel: w954 -> [w1542]
      tunnel: w953 -> [w1543]
      tunnel: w952 -> [w1544]
      tunnel: [w1544] -> w1104
      tunnel: [w1543] -> w1103
      tunnel: [w1542] -> w1102
      tunnel: [w1541] -> w1101
      tunnel: [w1547] -> w687
      tunnel: [w1550] -> w948
      tunnel: [w1549] -> w949
      tunnel: [w1548] -> w877
      tunnel: w1104 -> [w1553]
      tunnel: w1103 -> [w1552]
      tunnel: w1102 -> [w1551]
      tunnel: w1101 -> [w1546]
      tunnel: [w1545] -> w731
      frame #0 {
        # "Write Data"
        n197 = To Single Precision Float(number="Capacitance (uF)") -> (single precision float=w1540:sgl)
        n198 = To Variant(anything=w1540) -> (Variant=w1541:variant)
      }
      frame #1 {
        # "Resolve To TC"
        n199 = call <userlib>:"Resolve To TC Type.vi"("Handle"=w1551, "TypHdl"=w1552, "WData"=w1546, "error in"=w1553) -> ("Handle"=w1549:u32, "TypHdl"=w1550:u32, "bHasMatched"=w1545:bool, "ADSWData"=w1548:variant, "error out"=w1547:errorcluster)  [unwired: 7 in]
      }
    }
    n200 = flat-sequence {
      tunnel: w930 -> [w1512]
      tunnel: w929 -> [w1513]
      tunnel: w928 -> [w1514]
      tunnel: [w1514] -> w1096
      tunnel: [w1513] -> w1095
      tunnel: [w1512] -> w1094
      tunnel: [w1511] -> w1093
      tunnel: w792 -> [w1509]
      tunnel: [w1517] -> w681
      tunnel: [w1520] -> w924
      tunnel: [w1519] -> w925
      tunnel: [w1518] -> w875
      tunnel: w1096 -> [w1523]
      tunnel: w1095 -> [w1522]
      tunnel: w1094 -> [w1521]
      tunnel: w1093 -> [w1516]
      tunnel: [w1515] -> w735
      frame #0 {
        # "Write Data"
        n201 = To Long Integer(number=w1509) -> (32bit integer=w1510:i32)
        n202 = To Variant(anything=w1510) -> (Variant=w1511:variant)
      }
      frame #1 {
        # "Resolve To TC"
        n203 = call <userlib>:"Resolve To TC Type.vi"("Handle"=w1521, "TypHdl"=w1522, "WData"=w1516, "error in"=w1523) -> ("Handle"=w1519:u32, "TypHdl"=w1520:u32, "bHasMatched"=w1515:bool, "ADSWData"=w1518:variant, "error out"=w1517:errorcluster)  [unwired: 7 in]
      }
    }
    n204 = flat-sequence {
      tunnel: w962 -> [w1558]
      tunnel: [w1556] -> _
      tunnel: w960 -> [w1559]
      tunnel: [w1559] -> w1108
      tunnel: [w1556] -> w1107
      tunnel: [w1558] -> w1106
      tunnel: [w1557] -> w1105
      tunnel: w961 -> [w1556]
      tunnel: [w1562] -> w690
      tunnel: [w1565] -> w964
      tunnel: [w1564] -> w963
      tunnel: [w1563] -> w878
      tunnel: w1108 -> [w1568]
      tunnel: w1107 -> [w1567]
      tunnel: w1106 -> [w1566]
      tunnel: w1105 -> [w1561]
      tunnel: [w1560] -> w729
      frame #0 {
        # "Write Data"
        n205 = To Long Integer(number="Cycle Time (Sec)") -> (32bit integer=w1555:i32)
        n206 = To Variant(anything=w1555) -> (Variant=w1557:variant)
      }
      frame #1 {
        # "Resolve To TC"
        n207 = call <userlib>:"Resolve To TC Type.vi"("Handle"=w1566, "TypHdl"=w1567, "WData"=w1561, "error in"=w1568) -> ("Handle"=w1564:u32, "TypHdl"=w1565:u32, "bHasMatched"=w1560:bool, "ADSWData"=w1563:variant, "error out"=w1562:errorcluster)  [unwired: 7 in]
      }
    }
    n208 = flat-sequence {
      tunnel: w942 -> [w1527]
      tunnel: w941 -> [w1528]
      tunnel: w940 -> [w1529]
      tunnel: [w1529] -> w1100
      tunnel: [w1528] -> w1099
      tunnel: [w1527] -> w1098
      tunnel: [w1526] -> w1097
      tunnel: [w1532] -> w684
      tunnel: [w1535] -> w936
      tunnel: [w1534] -> w937
      tunnel: [w1533] -> w876
      tunnel: w1100 -> [w1538]
      tunnel: w1099 -> [w1537]
      tunnel: w1098 -> [w1536]
      tunnel: w1097 -> [w1531]
      tunnel: [w1530] -> w733
      frame #0 {
        # "Write Data"
        n209 = To Long Integer(number="Target Charge Volt (V) - Min 1500V - TEMPORARY LIMIT 12kV") -> (32bit integer=w1525:i32)
        n210 = To Variant(anything=w1525) -> (Variant=w1526:variant)
      }
      frame #1 {
        # "Resolve To TC"
        n211 = call <userlib>:"Resolve To TC Type.vi"("Handle"=w1536, "TypHdl"=w1537, "WData"=w1531, "error in"=w1538) -> ("Handle"=w1534:u32, "TypHdl"=w1535:u32, "bHasMatched"=w1530:bool, "ADSWData"=w1533:variant, "error out"=w1532:errorcluster)  [unwired: 7 in]
      }
    }
    n212 = flat-sequence {
      tunnel: w918 -> [w1497]
      tunnel: w917 -> [w1498]
      tunnel: w916 -> [w1499]
      tunnel: [w1499] -> w1092
      tunnel: [w1498] -> w1091
      tunnel: [w1497] -> w1090
      tunnel: [w1496] -> w1089
      tunnel: [w1502] -> w678
      tunnel: [w1505] -> w912
      tunnel: [w1504] -> w913
      tunnel: [w1503] -> w874
      tunnel: w1092 -> [w1508]
      tunnel: w1091 -> [w1507]
      tunnel: w1090 -> [w1506]
      tunnel: w1089 -> [w1501]
      tunnel: [w1500] -> w737
      frame #0 {
        # "Write Data"
        n213 = To Single Precision Float(number="Hold Time Before Shot (seconds)") -> (single precision float=w1495:sgl)
        n214 = To Variant(anything=w1495) -> (Variant=w1496:variant)
      }
      frame #1 {
        # "Resolve To TC"
        n215 = call <userlib>:"Resolve To TC Type.vi"("Handle"=w1506, "TypHdl"=w1507, "WData"=w1501, "error in"=w1508) -> ("Handle"=w1504:u32, "TypHdl"=w1505:u32, "bHasMatched"=w1500:bool, "ADSWData"=w1503:variant, "error out"=w1502:errorcluster)  [unwired: 7 in]
      }
    }
    n216 = flat-sequence {
      tunnel: w978 -> [w1392]
      tunnel: w977 -> [w1393]
      tunnel: w976 -> [w1394]
      tunnel: [w1394] -> w1064
      tunnel: [w1393] -> w1063
      tunnel: [w1392] -> w1062
      tunnel: [w1391] -> w1061
      tunnel: [w1397] -> w692
      tunnel: [w1400] -> w972
      tunnel: [w1399] -> w973
      tunnel: [w1398] -> w879
      tunnel: w1064 -> [w1403]
      tunnel: w1063 -> [w1402]
      tunnel: w1062 -> [w1401]
      tunnel: w1061 -> [w1396]
      tunnel: [w1395] -> w728
      frame #0 {
        # "Write Data"
        n217 = And(x="CLEAR FAULT", y="CLEAR FAULT") -> (x .and. y?=w1390:bool)
        n218 = To Variant(anything=w1390) -> (Variant=w1391:variant)
      }
      frame #1 {
        # "Resolve To TC"
        n219 = call <userlib>:"Resolve To TC Type.vi"("Handle"=w1401, "TypHdl"=w1402, "WData"=w1396, "error in"=w1403) -> ("Handle"=w1399:u32, "TypHdl"=w1400:u32, "bHasMatched"=w1395:bool, "ADSWData"=w1398:variant, "error out"=w1397:errorcluster)  [unwired: 7 in]
      }
    }
    n220 = flat-sequence {
      tunnel: w1026 -> [w1452]
      tunnel: w1025 -> [w1453]
      tunnel: w1024 -> [w1454]
      tunnel: [w1454] -> w1080
      tunnel: [w1453] -> w1079
      tunnel: [w1452] -> w1078
      tunnel: [w1451] -> w1077
      tunnel: [w1457] -> w704
      tunnel: [w1460] -> w1020
      tunnel: [w1459] -> w1021
      tunnel: [w1458] -> w883
      tunnel: w1080 -> [w1463]
      tunnel: w1079 -> [w1462]
      tunnel: w1078 -> [w1461]
      tunnel: w1077 -> [w1456]
      tunnel: [w1455] -> w720
      frame #0 {
        # "Write Data"
        n221 = And(x="Hold", y="Hold") -> (x .and. y?=w1450:bool)
        n222 = To Variant(anything=w1450) -> (Variant=w1451:variant)
      }
      frame #1 {
        # "Resolve To TC"
        n223 = call <userlib>:"Resolve To TC Type.vi"("Handle"=w1461, "TypHdl"=w1462, "WData"=w1456, "error in"=w1463) -> ("Handle"=w1459:u32, "TypHdl"=w1460:u32, "bHasMatched"=w1455:bool, "ADSWData"=w1458:variant, "error out"=w1457:errorcluster)  [unwired: 7 in]
      }
    }
    n224 = flat-sequence {
      tunnel: w1002 -> [w1422]
      tunnel: w1001 -> [w1423]
      tunnel: w1000 -> [w1424]
      tunnel: [w1424] -> w1072
      tunnel: [w1423] -> w1071
      tunnel: [w1422] -> w1070
      tunnel: [w1421] -> w1069
      tunnel: [w1427] -> w698
      tunnel: [w1430] -> w996
      tunnel: [w1429] -> w997
      tunnel: [w1428] -> w881
      tunnel: w1072 -> [w1433]
      tunnel: w1071 -> [w1432]
      tunnel: w1070 -> [w1431]
      tunnel: w1069 -> [w1426]
      tunnel: [w1425] -> w724
      frame #0 {
        # "Write Data"
        n225 = And(x="Shot", y="Shot") -> (x .and. y?=w1420:bool)
        n226 = To Variant(anything=w1420) -> (Variant=w1421:variant)
      }
      frame #1 {
        # "Resolve To TC"
        n227 = call <userlib>:"Resolve To TC Type.vi"("Handle"=w1431, "TypHdl"=w1432, "WData"=w1426, "error in"=w1433) -> ("Handle"=w1429:u32, "TypHdl"=w1430:u32, "bHasMatched"=w1425:bool, "ADSWData"=w1428:variant, "error out"=w1427:errorcluster)  [unwired: 7 in]
      }
    }
    n228 = flat-sequence {
      tunnel: w1034 -> [w1468]
      tunnel: [w1464] -> _
      tunnel: w1032 -> [w1469]
      tunnel: [w1469] -> w1084
      tunnel: [w1464] -> w1083
      tunnel: [w1468] -> w1082
      tunnel: [w1467] -> w1081
      tunnel: w1033 -> [w1464]
      tunnel: [w1472] -> w707
      tunnel: [w1475] -> w1036
      tunnel: [w1474] -> w1035
      tunnel: [w1473] -> w884
      tunnel: w1084 -> [w1478]
      tunnel: w1083 -> [w1477]
      tunnel: w1082 -> [w1476]
      tunnel: w1081 -> [w1471]
      tunnel: [w1470] -> w718
      frame #0 {
        # "Write Data"
        n229 = And(x="Manual/Auto", y="Manual/Auto") -> (x .and. y?=w1466:bool)
        n230 = To Variant(anything=w1466) -> (Variant=w1467:variant)
      }
      frame #1 {
        # "Resolve To TC"
        n231 = call <userlib>:"Resolve To TC Type.vi"("Handle"=w1476, "TypHdl"=w1477, "WData"=w1471, "error in"=w1478) -> ("Handle"=w1474:u32, "TypHdl"=w1475:u32, "bHasMatched"=w1470:bool, "ADSWData"=w1473:variant, "error out"=w1472:errorcluster)  [unwired: 7 in]
      }
    }
    n232 = flat-sequence {
      tunnel: w1014 -> [w1437]
      tunnel: w1013 -> [w1438]
      tunnel: w1012 -> [w1439]
      tunnel: [w1439] -> w1076
      tunnel: [w1438] -> w1075
      tunnel: [w1437] -> w1074
      tunnel: [w1436] -> w1073
      tunnel: [w1442] -> w701
      tunnel: [w1445] -> w1008
      tunnel: [w1444] -> w1009
      tunnel: [w1443] -> w882
      tunnel: w1076 -> [w1448]
      tunnel: w1075 -> [w1447]
      tunnel: w1074 -> [w1446]
      tunnel: w1073 -> [w1441]
      tunnel: [w1440] -> w722
      frame #0 {
        # "Write Data"
        n233 = And(x="Charge", y="Charge") -> (x .and. y?=w1435:bool)
        n234 = To Variant(anything=w1435) -> (Variant=w1436:variant)
      }
      frame #1 {
        # "Resolve To TC"
        n235 = call <userlib>:"Resolve To TC Type.vi"("Handle"=w1446, "TypHdl"=w1447, "WData"=w1441, "error in"=w1448) -> ("Handle"=w1444:u32, "TypHdl"=w1445:u32, "bHasMatched"=w1440:bool, "ADSWData"=w1443:variant, "error out"=w1442:errorcluster)  [unwired: 7 in]
      }
    }
    n236 = flat-sequence {
      tunnel: w990 -> [w1407]
      tunnel: w989 -> [w1408]
      tunnel: w988 -> [w1409]
      tunnel: [w1409] -> w1068
      tunnel: [w1408] -> w1067
      tunnel: [w1407] -> w1066
      tunnel: [w1406] -> w1065
      tunnel: [w1412] -> w695
      tunnel: [w1415] -> w984
      tunnel: [w1414] -> w985
      tunnel: [w1413] -> w880
      tunnel: w1068 -> [w1418]
      tunnel: w1067 -> [w1417]
      tunnel: w1066 -> [w1416]
      tunnel: w1065 -> [w1411]
      tunnel: [w1410] -> w726
      frame #0 {
        # "Write Data"
        n237 = And(x="HV Switch Mode", y="HV Switch Mode") -> (x .and. y?=w1405:bool)
        n238 = To Variant(anything=w1405) -> (Variant=w1406:variant)
      }
      frame #1 {
        # "Resolve To TC"
        n239 = call <userlib>:"Resolve To TC Type.vi"("Handle"=w1416, "TypHdl"=w1417, "WData"=w1411, "error in"=w1418) -> ("Handle"=w1414:u32, "TypHdl"=w1415:u32, "bHasMatched"=w1410:bool, "ADSWData"=w1413:variant, "error out"=w1412:errorcluster)  [unwired: 7 in]
      }
    }
    n240 = flat-sequence {
      tunnel: w1050 -> [w1338]
      tunnel: w1049 -> [w1339]
      tunnel: w1048 -> [w1340]
      tunnel: [w1340] -> w783
      tunnel: [w1339] -> w782
      tunnel: [w1338] -> w781
      tunnel: [w1337] -> w780
      tunnel: w783 -> [w1349]
      tunnel: w782 -> [w1348]
      tunnel: w781 -> [w1347]
      tunnel: w780 -> [w1342]
      tunnel: [w1343] -> w710
      tunnel: [w1346] -> w1044
      tunnel: [w1345] -> w1045
      tunnel: [w1344] -> w779
      tunnel: [w1341] -> w716
      frame #0 {
        # "Write Data"
        n241 = And(x="STOP", y="STOP") -> (x .and. y?=w1336:bool)
        n242 = To Variant(anything=w1336) -> (Variant=w1337:variant)
      }
      frame #1 {
        # "Resolve To TC"
        n243 = call <userlib>:"Resolve To TC Type.vi"("Handle"=w1347, "TypHdl"=w1348, "WData"=w1342, "error in"=w1349) -> ("Handle"=w1345:u32, "TypHdl"=w1346:u32, "bHasMatched"=w1341:bool, "ADSWData"=w1344:variant, "error out"=w1343:errorcluster)  [unwired: 7 in]
      }
    }
    n244 = flat-sequence {
      tunnel: w661 -> [w1285]
      tunnel: w660 -> [w1281]
      tunnel: w659 -> [w1286]
      tunnel: [w1286] -> w670
      tunnel: [w1281] -> w669
      tunnel: [w1285] -> w668
      tunnel: [w1284] -> w667
      tunnel: [w1289] -> w480
      tunnel: [w1292] -> w654
      tunnel: [w1291] -> w655
      tunnel: [w1290] -> w658
      tunnel: w670 -> [w1295]
      tunnel: w669 -> [w1294]
      tunnel: w668 -> [w1293]
      tunnel: w667 -> [w1288]
      tunnel: [w1287] -> w652
      frame #0 {
        # "Write Data"
        n245 = And(x="Reset Test Number", y="Reset Test Number") -> (x .and. y?=w1283:bool)
        n246 = To Variant(anything=w1283) -> (Variant=w1284:variant)
      }
      frame #1 {
        # "Resolve To TC"
        n247 = call <userlib>:"Resolve To TC Type.vi"("Handle"=w1293, "TypHdl"=w1294, "WData"=w1288, "error in"=w1295) -> ("Handle"=w1291:u32, "TypHdl"=w1292:u32, "bHasMatched"=w1287:bool, "ADSWData"=w1290:variant, "error out"=w1289:errorcluster)  [unwired: 7 in]
      }
    }
    n248 = flat-sequence {
      tunnel: w1060 -> [w1304]
      tunnel: w1059 -> [w1305]
      tunnel: w1056 -> [w1306]
      tunnel: [w1306] -> w778
      tunnel: [w1305] -> w777
      tunnel: [w1304] -> w776
      tunnel: [w1303] -> w775
      tunnel: [w1301] -> _
      tunnel: [w1301] -> w774
      tunnel: w791 -> [w1301]
      tunnel: w790 -> [w1300]
      tunnel: [w1300] -> w773
      tunnel: w789 -> [w1299]
      tunnel: [w1299] -> w772
      tunnel: w788 -> [w1298]
      tunnel: [w1298] -> w771
      tunnel: w787 -> [w1297]
      tunnel: [w1297] -> w770
      tunnel: ["START"] -> w574
      tunnel: w778 -> [w1320]
      tunnel: w777 -> [w1319]
      tunnel: w776 -> [w1318]
      tunnel: w775 -> [w1313]
      tunnel: [w1314] -> w769
      tunnel: [w1317] -> w768
      tunnel: [w1316] -> w767
      tunnel: [w1315] -> w766
      tunnel: [w1312] -> w765
      tunnel: w774 -> [w1311]
      tunnel: [w1311] -> w764
      tunnel: w773 -> [w1310]
      tunnel: [w1310] -> w763
      tunnel: w772 -> [w1309]
      tunnel: [w1309] -> w762
      tunnel: w771 -> [w1308]
      tunnel: [w1308] -> w761
      tunnel: [w1307] -> w760
      tunnel: w770 -> [w1307]
      tunnel: [w1331] -> w743
      tunnel: [w1332] -> w1058
      tunnel: [w1333] -> w1057
      tunnel: [w1334] -> w713
      tunnel: w769 -> [w1334]
      tunnel: w768 -> [w1333]
      tunnel: w767 -> [w1332]
      tunnel: w766 -> [w1323]
      tunnel: w765 -> [w1331]
      tunnel: w764 -> [w1330]
      tunnel: w763 -> [w1329]
      tunnel: w762 -> [w1328]
      tunnel: w761 -> [w1327]
      tunnel: w760 -> [w1326]
      tunnel: [w1325] -> w786
      tunnel: [w1324] -> w785
      tunnel: [w1322] -> w714
      tunnel: [w1321] -> w758
      frame #0 {
        # "Write Data"
        n249 = And(x="START", y="START") -> (x .and. y?=w1302:bool)
        n250 = To Variant(anything=w1302) -> (Variant=w1303:variant)
      }
      frame #1 {
        # "Resolve To TC"
        n251 = call <userlib>:"Resolve To TC Type.vi"("Handle"=w1318, "TypHdl"=w1319, "WData"=w1313, "error in"=w1320) -> ("Handle"=w1316:u32, "TypHdl"=w1317:u32, "bHasMatched"=w1312:bool, "ADSWData"=w1315:variant, "error out"=w1314:errorcluster)  [unwired: 7 in]
      }
      frame #2 {
        # "Write"
        n252 = call <userlib>:"Send Writer-Request.vi"("Handle"=w1330, "SymbolName"=w1329, "WriterMode"=w1328, "WriteHandle"=w1327, "error constant"=w1326, "ADS Write Data"=w1323) -> ("Handle"=w1325:u32, "WriteHandle"=w1324:u32, "Write status?"=w1321:bool, "error IO"=w1322:errorcluster)  [unwired: 5 in, 1 out]
      }
    }
    n253 = To Single Precision Float(number="Duty Cycle") -> (single precision float=w531:sgl)
    n254 = And(x="Voltage Held by PSU", y="Voltage Held by PSU") -> (x .and. y?=w517:bool)
    n255 = And(x="Current Control", y="Current Control") -> (x .and. y?=w538:bool)
    n256 = To Variant(anything=w531) -> (Variant=w535:variant)
    n257 = And(x="Dump", y="Dump") -> (x .and. y?=w547:bool)
    n258 = To Variant(anything=w517) -> (Variant=w515:variant)
    n259 = To Variant(anything=w538) -> (Variant=w536:variant)
    n260 = To Variant(anything=w547) -> (Variant=w548:variant)
    n261 = call-poly <userlib>:"Write TypeResolved.vi"("Handle"=w518, "SymbolName"=w519, "WData"=w515, "error constant"=w514) -> ("Write Status?"=w507:bool, "Has Matched?"=w508:bool, "error out"=w513:errorcluster)  [unwired: 8 in, 1 out]
    n262 = flat-sequence {
      tunnel: w899 -> [w1700]
      tunnel: w898 -> [w1698]
      tunnel: w897 -> [w1696]
      tunnel: [w1699] -> w1143
      tunnel: [w1697] -> w1142
      tunnel: [w1695] -> w1141
      tunnel: [w1694] -> w1140
      tunnel: [w1693] -> w1139
      tunnel: [w1692] -> w1138
      tunnel: [w1691] -> w1137
      tunnel: [w1690] -> w1136
      tunnel: [w1689] -> w1135
      tunnel: [w1688] -> w1134
      tunnel: [w1687] -> w1133
      tunnel: w895 -> [w1686]
      tunnel: w894 -> [w1685]
      tunnel: w893 -> [w1684]
      tunnel: w892 -> [w1683]
      tunnel: w891 -> [w1682]
      tunnel: w890 -> [w1681]
      tunnel: [w1680] -> w1132
      tunnel: [w1679] -> w1131
      tunnel: [w1678] -> w1130
      tunnel: [w1677] -> w1129
      tunnel: [w1676] -> w1128
      tunnel: [w1675] -> w1127
      tunnel: [w1674] -> w1126
      tunnel: [w1673] -> w1125
      tunnel: [w1672] -> w1124
      tunnel: [w1671] -> w1123
      tunnel: [w1670] -> w1122
      tunnel: [w1669] -> w1121
      tunnel: [w1668] -> w1120
      tunnel: [w1667] -> w1119
      tunnel: [w1666] -> w1118
      tunnel: [w1665] -> w1117
      tunnel: [w1664] -> w1116
      tunnel: [w1663] -> w1115
      tunnel: [w1662] -> w1114
      tunnel: [w1661] -> w1113
      tunnel: [w1660] -> w1112
      tunnel: [w1659] -> w1111
      tunnel: [w1658] -> w1110
      tunnel: [w1657] -> w1109
      tunnel: w856 -> [w1656]
      tunnel: [w1655] -> w855
      tunnel: [w1654] -> w854
      tunnel: [w1653] -> w853
      tunnel: [w1652] -> w852
      tunnel: [w1651] -> w851
      tunnel: w849 -> [w1570]
      tunnel: [w1650] -> w848
      tunnel: w846 -> [w1649]
      tunnel: [w1648] -> w845
      tunnel: [w1647] -> w844
      tunnel: [w1646] -> w843
      tunnel: w842 -> [w1645]
      tunnel: w841 -> [w1644]
      tunnel: [w1643] -> w840
      tunnel: [w1642] -> w839
      tunnel: [w1641] -> w838
      tunnel: [w1640] -> w837
      tunnel: [w1639] -> w836
      tunnel: [w1638] -> w835
      tunnel: [w1637] -> w834
      tunnel: [w1636] -> w833
      tunnel: w825 -> [w1635]
      tunnel: w824 -> [w1634]
      tunnel: w823 -> [w1633]
      tunnel: [w1632] -> w822
      tunnel: [w1631] -> w821
      tunnel: [w1630] -> w820
      tunnel: [w1629] -> w819
      tunnel: [w1628] -> w818
      tunnel: [w1627] -> w817
      tunnel: [w1626] -> w816
      tunnel: [w1625] -> w815
      tunnel: [w1624] -> w814
      tunnel: [w1623] -> w813
      tunnel: [w1622] -> w812
      tunnel: [w1621] -> w811
      tunnel: [w1574] -> _
      tunnel: w784 -> [w1574]
      tunnel: [w1620] -> w626
      tunnel: [w1619] -> w625
      tunnel: [w1618] -> w624
      tunnel: w623 -> [w1617]
      tunnel: [w1616] -> w619
      tunnel: w617 -> [w1615]
      tunnel: [w1614] -> w616
      tunnel: [w1613] -> w615
      tunnel: [w1612] -> w614
      tunnel: [w1611] -> w613
      tunnel: w612 -> [w1610]
      tunnel: w611 -> [w1609]
      tunnel: w610 -> [w1608]
      tunnel: [w1607] -> w609
      tunnel: [w1606] -> w608
      tunnel: [w1605] -> w606
      tunnel: [w1604] -> w604
      tunnel: [w1603] -> w603
      tunnel: [w1602] -> w602
      tunnel: [w1601] -> w601
      tunnel: [w1600] -> w598
      tunnel: w597 -> [w1599]
      tunnel: [w1598] -> w596
      tunnel: [w1597] -> w595
      tunnel: [w1596] -> w594
      tunnel: w572 -> [w1595]
      tunnel: w571 -> [w1594]
      tunnel: [w1593] -> w570
      tunnel: [w1592] -> w569
      tunnel: [w1591] -> w568
      tunnel: [w1590] -> w567
      tunnel: [w1589] -> w566
      tunnel: [w1588] -> w565
      tunnel: w564 -> [w1587]
      tunnel: [w1586] -> w563
      tunnel: [w1585] -> w562
      tunnel: [w1584] -> w561
      tunnel: w545 -> [w1583]
      tunnel: [w1582] -> w544
      tunnel: [w1581] -> w543
      tunnel: [w1580] -> w542
      tunnel: [w1579] -> w502
      tunnel: [w1578] -> w501
      tunnel: w500 -> [w1577]
      tunnel: w499 -> [w1575]
      tunnel: [w1576] -> w498
      tunnel: [w1573] -> w497
      tunnel: [w1572] -> w496
      tunnel: [w1571] -> w495
      tunnel: [w1569] -> w482
      tunnel: w1143 -> [w1913]
      tunnel: w1142 -> [w1926]
      tunnel: w1141 -> [_]
      tunnel: w1140 -> [w1912]
      tunnel: w1139 -> [w1911]
      tunnel: w1138 -> [w1738]
      tunnel: [w1839] -> w896
      tunnel: w1137 -> [w1925]
      tunnel: w1136 -> [w1927]
      tunnel: w1135 -> [w1929]
      tunnel: w1134 -> [w1747]
      tunnel: w1133 -> [_]
      tunnel: w1132 -> [w1908]
      tunnel: w1131 -> [w1923]
      tunnel: w1130 -> [w1921]
      tunnel: w1129 -> [w1919]
      tunnel: w1128 -> [w1917]
      tunnel: w1127 -> [w1915]
      tunnel: [w1852] -> w889
      tunnel: w1126 -> [w1907]
      tunnel: w1125 -> [w1906]
      tunnel: w1124 -> [w1905]
      tunnel: w1123 -> [w1904]
      tunnel: w1122 -> [w1903]
      tunnel: w1121 -> [w1902]
      tunnel: w1120 -> [_]
      tunnel: w1119 -> [w1736]
      tunnel: w1118 -> [_]
      tunnel: w1117 -> [w1734]
      tunnel: w1116 -> [_]
      tunnel: w1115 -> [w1732]
      tunnel: w1114 -> [_]
      tunnel: w1113 -> [w1730]
      tunnel: w1112 -> [_]
      tunnel: w1111 -> [w1728]
      tunnel: w1110 -> [_]
      tunnel: w1109 -> [w1726]
      tunnel: [w1854] -> w888
      tunnel: [w1856] -> w887
      tunnel: [w1858] -> w886
      tunnel: [w1860] -> w885
      tunnel: w855 -> [w1724]
      tunnel: w854 -> [w1893]
      tunnel: w853 -> [_]
      tunnel: w852 -> [w1823]
      tunnel: w851 -> [w1888]
      tunnel: [w1843] -> w850
      tunnel: w848 -> [w1892]
      tunnel: [w1841] -> w847
      tunnel: w845 -> [w1891]
      tunnel: w844 -> [w1889]
      tunnel: w843 -> [_]
      tunnel: w840 -> [w1885]
      tunnel: w839 -> [w1884]
      tunnel: w838 -> [w1881]
      tunnel: w837 -> [w1880]
      tunnel: w836 -> [w1879]
      tunnel: w835 -> [w1878]
      tunnel: w834 -> [_]
      tunnel: w833 -> [_]
      tunnel: [w1845] -> w832
      tunnel: [w1847] -> w831
      tunnel: [w1862] -> w828
      tunnel: [w1865] -> w827
      tunnel: [w1864] -> w826
      tunnel: w822 -> [w1876]
      tunnel: w821 -> [w1874]
      tunnel: w820 -> [w1872]
      tunnel: w819 -> [w1742]
      tunnel: w818 -> [w1740]
      tunnel: w817 -> [w1744]
      tunnel: w816 -> [w1871]
      tunnel: w815 -> [w1870]
      tunnel: w814 -> [w1869]
      tunnel: w813 -> [_]
      tunnel: w812 -> [_]
      tunnel: w811 -> [_]
      tunnel: [w1850] -> w810
      tunnel: [w1848] -> w809
      tunnel: [w1837] -> w808
      tunnel: [w1838] -> _
      tunnel: [w1829] -> w671
      tunnel: [w1831] -> w627
      tunnel: w626 -> [w1746]
      tunnel: w625 -> [w1834]
      tunnel: w624 -> [_]
      tunnel: [w1832] -> w622
      tunnel: w619 -> [w1826]
      tunnel: w616 -> [w1821]
      tunnel: w615 -> [w1818]
      tunnel: w614 -> [w1816]
      tunnel: w613 -> [w1803]
      tunnel: w609 -> [w1722]
      tunnel: w608 -> [w1815]
      tunnel: [w1814] -> w607
      tunnel: w606 -> [w1813]
      tunnel: [w1812] -> w605
      tunnel: w604 -> [w1811]
      tunnel: w603 -> [w1718]
      tunnel: w602 -> [w1810]
      tunnel: w601 -> [w1716]
      tunnel: [w1809] -> w600
      tunnel: [w1808] -> w599
      tunnel: w598 -> [w1720]
      tunnel: [w1807] -> w581
      tunnel: [w1806] -> w579
      tunnel: [w1805] -> w589
      tunnel: w596 -> [w1798]
      tunnel: w595 -> [w1714]
      tunnel: w594 -> [w1801]
      tunnel: [w1800] -> w593
      tunnel: w570 -> [w1794]
      tunnel: w569 -> [w1712]
      tunnel: w568 -> [w1796]
      tunnel: w567 -> [w1795]
      tunnel: w566 -> [w1790]
      tunnel: w565 -> [w1710]
      tunnel: w563 -> [w1776]
      tunnel: w562 -> [w1708]
      tunnel: w561 -> [w1789]
      tunnel: [w1782] -> w560
      tunnel: [w1781] -> w559
      tunnel: [w1780] -> w558
      tunnel: [w1779] -> w557
      tunnel: w544 -> [w1757]
      tunnel: w543 -> [w1774]
      tunnel: w542 -> [w1706]
      tunnel: [w1773] -> w541
      tunnel: w502 -> [w1704]
      tunnel: w501 -> [w1758]
      tunnel: w498 -> [w1753]
      tunnel: w497 -> [w1755]
      tunnel: w496 -> [w1754]
      tunnel: w495 -> [w1702]
      tunnel: [w1749] -> w494
      tunnel: [w1748] -> w493
      tunnel: w482 -> [_]
      frame #0 {
        # "Read and Resolve Data."
        # "Read/Resolve Symbol N"
        # "Read Data and Resolve Type"
        n263 = call-poly <userlib>:"Read TypeResolved.vi"("Handle"=w1574, "SymbolName"=w1644, "error constant"=w1570) -> ("Handle"=w1637:u32, "Read Status?"=w1642:bool, "RData"=w1638:variant, "error out"=w1641:errorcluster)  [unwired: 9 in]
        n264 = call-poly <userlib>:"Read TypeResolved.vi"("Handle"=w1574, "SymbolName"=w1645, "error constant"=w1570) -> ("Handle"=w1636:u32, "Read Status?"=w1643:bool, "RData"=w1639:variant, "error out"=w1640:errorcluster)  [unwired: 9 in]
        n265 = call-poly <userlib>:"Read TypeResolved.vi"("Handle"=w1574, "SymbolName"=w1698, "error constant"=w1570) -> ("Handle"=w1688:u32, "Read Status?"=w1690:bool, "RData"=w1694:variant, "error out"=w1699:errorcluster)  [unwired: 9 in]
        n266 = call-poly <userlib>:"Read TypeResolved.vi"("Handle"=w1574, "SymbolName"=w1649, "error constant"=w1570) -> ("Handle"=w1646:u32, "Read Status?"=w1648:bool, "RData"=w1647:variant, "error out"=w1651:errorcluster)  [unwired: 9 in]
        n267 = call-poly <userlib>:"Read TypeResolved.vi"("Handle"=w1574, "SymbolName"=w1700, "error constant"=w1570) -> ("Handle"=w1687:u32, "Read Status?"=w1689:bool, "RData"=w1693:variant, "error out"=w1650:errorcluster)  [unwired: 9 in]
        n268 = call-poly <userlib>:"Read TypeResolved.vi"("Handle"=w1574, "SymbolName"=w1577, "error constant"=w1570) -> ("Read Status?"=w1576:bool, "RData"=w1579:variant, "error out"=w1578:errorcluster)  [unwired: 9 in, 1 out]
        n269 = call-poly <userlib>:"Read TypeResolved.vi"("Handle"=w1574, "SymbolName"=w1696, "error constant"=w1570) -> ("Handle"=w1695:u32, "Read Status?"=w1691:bool, "RData"=w1692:variant, "error out"=w1697:errorcluster)  [unwired: 9 in]
        n270 = call-poly <userlib>:"Read TypeResolved.vi"("Handle"=w1574, "SymbolName"=w1686, "error constant"=w1570) -> ("Handle"=w1668:u32, "Read Status?"=w1675:bool, "RData"=w1667:variant, "error out"=w1674:errorcluster)  [unwired: 9 in]
        n271 = call-poly <userlib>:"Read TypeResolved.vi"("Handle"=w1574, "SymbolName"=w1587, "error constant"=w1570) -> ("Read Status?"=w1586:bool, "RData"=w1585:variant, "error out"=w1584:errorcluster)  [unwired: 9 in, 1 out]
        n272 = call-poly <userlib>:"Read TypeResolved.vi"("Handle"=w1574, "SymbolName"=w1575, "error constant"=w1570) -> ("Read Status?"=w1572:bool, "RData"=w1571:variant, "error out"=w1573:errorcluster)  [unwired: 9 in, 1 out]
        n273 = call-poly <userlib>:"Read TypeResolved.vi"("Handle"=w1574, "SymbolName"=w1583, "error constant"=w1570) -> ("Read Status?"=w1582:bool, "RData"=w1580:variant, "error out"=w1581:errorcluster)  [unwired: 9 in, 1 out]
        n274 = call-poly <userlib>:"Read TypeResolved.vi"("Handle"=w1574, "SymbolName"=w1684, "error constant"=w1570) -> ("Handle"=w1664:u32, "Read Status?"=w1677:bool, "RData"=w1663:variant, "error out"=w1672:errorcluster)  [unwired: 9 in]
        n275 = call-poly <userlib>:"Read TypeResolved.vi"("Handle"=w1574, "SymbolName"=w1682, "error constant"=w1570) -> ("Handle"=w1660:u32, "Read Status?"=w1679:bool, "RData"=w1659:variant, "error out"=w1670:errorcluster)  [unwired: 9 in]
        n276 = call-poly <userlib>:"Read TypeResolved.vi"("Handle"=w1574, "SymbolName"=w1599, "error constant"=w1570) -> ("Read Status?"=w1598:bool, "RData"=w1597:variant, "error out"=w1596:errorcluster)  [unwired: 9 in, 1 out]
        n277 = call-poly <userlib>:"Read TypeResolved.vi"("Handle"=w1574, "SymbolName"=w1595, "error constant"=w1570) -> ("Read Status?"=w1593:bool, "RData"=w1592:variant, "error out"=w1591:errorcluster)  [unwired: 9 in, 1 out]
        n278 = call-poly <userlib>:"Read TypeResolved.vi"("Handle"=w1574, "SymbolName"=w1594, "error constant"=w1570) -> ("Read Status?"=w1589:bool, "RData"=w1588:variant, "error out"=w1590:errorcluster)  [unwired: 9 in, 1 out]
        n279 = call-poly <userlib>:"Read TypeResolved.vi"("Handle"=w1574, "SymbolName"=w1685, "error constant"=w1570) -> ("Handle"=w1666:u32, "Read Status?"=w1676:bool, "RData"=w1665:variant, "error out"=w1673:errorcluster)  [unwired: 9 in]
        n280 = call-poly <userlib>:"Read TypeResolved.vi"("Handle"=w1574, "SymbolName"=w1683, "error constant"=w1570) -> ("Handle"=w1662:u32, "Read Status?"=w1678:bool, "RData"=w1661:variant, "error out"=w1671:errorcluster)  [unwired: 9 in]
        n281 = call-poly <userlib>:"Read TypeResolved.vi"("Handle"=w1574, "SymbolName"=w1681, "error constant"=w1570) -> ("Handle"=w1658:u32, "Read Status?"=w1680:bool, "RData"=w1657:variant, "error out"=w1669:errorcluster)  [unwired: 9 in]
        n282 = call-poly <userlib>:"Read TypeResolved.vi"("Handle"=w1574, "SymbolName"=w1656, "error constant"=w1570) -> ("Handle"=w1653:u32, "Read Status?"=w1652:bool, "RData"=w1655:variant, "error out"=w1654:errorcluster)  [unwired: 9 in]
        n283 = call-poly <userlib>:"Read TypeResolved.vi"("Handle"=w1574, "SymbolName"=w1615, "error constant"=w1570) -> ("Handle"=w1569:u32, "Read Status?"=w1614:bool, "RData"=w1607:variant, "error out"=w1606:errorcluster)  [unwired: 9 in]
        n284 = call-poly <userlib>:"Read TypeResolved.vi"("Handle"=w1574, "SymbolName"=w1610, "error constant"=w1570) -> ("Read Status?"=w1613:bool, "RData"=w1600:variant, "error out"=w1605:errorcluster)  [unwired: 9 in, 1 out]
        n285 = call-poly <userlib>:"Read TypeResolved.vi"("Handle"=w1574, "SymbolName"=w1608, "error constant"=w1570) -> ("Read Status?"=w1611:bool, "RData"=w1601:variant, "error out"=w1602:errorcluster)  [unwired: 9 in, 1 out]
        n286 = call-poly <userlib>:"Read TypeResolved.vi"("Handle"=w1574, "SymbolName"=w1609, "error constant"=w1570) -> ("Read Status?"=w1612:bool, "RData"=w1603:variant, "error out"=w1604:errorcluster)  [unwired: 9 in, 1 out]
        n287 = call-poly <userlib>:"Read TypeResolved.vi"("Handle"=w1574, "SymbolName"=w1635, "error constant"=w1570) -> ("Handle"=w1623:u32, "Read Status?"=w1632:bool, "RData"=w1628:variant, "error out"=w1624:errorcluster)  [unwired: 9 in]
        n288 = call-poly <userlib>:"Read TypeResolved.vi"("Handle"=w1574, "SymbolName"=w1634, "error constant"=w1570) -> ("Handle"=w1622:u32, "Read Status?"=w1631:bool, "RData"=w1629:variant, "error out"=w1625:errorcluster)  [unwired: 9 in]
        n289 = call-poly <userlib>:"Read TypeResolved.vi"("Handle"=w1574, "SymbolName"=w1617, "error constant"=w1570) -> ("Handle"=w1618:u32, "Read Status?"=w1616:bool, "RData"=w1620:variant, "error out"=w1619:errorcluster)  [unwired: 9 in]
        n290 = call-poly <userlib>:"Read TypeResolved.vi"("Handle"=w1574, "SymbolName"=w1633, "error constant"=w1570) -> ("Handle"=w1621:u32, "Read Status?"=w1630:bool, "RData"=w1627:variant, "error out"=w1626:errorcluster)  [unwired: 9 in]
      }
      frame #1 {
        # "Cast Symbol N to LabVIEW Type"
        # "Variant To Data"
        n291 = To Variant(anything=w1702) -> (Variant=w1701:variant)
        n292 = To Variant(anything=w1744) -> (Variant=w1743:variant)
        n293 = To Variant(anything=w1716) -> (Variant=w1715:variant)
        n294 = To Variant(anything=w1742) -> (Variant=w1741:variant)
        n295 = To Variant(anything=w1710) -> (Variant=w1709:variant)
        n296 = To Variant(anything=w1712) -> (Variant=w1711:variant)
        n297 = To Variant(anything=w1704) -> (Variant=w1703:variant)
        n298 = To Variant(anything=w1714) -> (Variant=w1713:variant)
        n299 = To Variant(anything=w1706) -> (Variant=w1705:variant)
        n300 = To Variant(anything=w1708) -> (Variant=w1707:variant)
        n301 = To Variant(anything=w1740) -> (Variant=w1739:variant)
        n302 = To Variant(anything=w1724) -> (Variant=w1723:variant)
        n303 = To Variant(anything=w1722) -> (Variant=w1721:variant)
        n304 = To Variant(anything=w1720) -> (Variant=w1719:variant)
        n305 = To Variant(anything=w1734) -> (Variant=w1733:variant)
        n306 = To Variant(anything=w1718) -> (Variant=w1717:variant)
        n307 = To Variant(anything=w1738) -> (Variant=w1737:variant)
        n308 = To Variant(anything=w1736) -> (Variant=w1735:variant)
        n309 = To Variant(anything=w1726) -> (Variant=w1725:variant)
        n310 = To Variant(anything=w1746) -> (Variant=w1745:variant)
        n311 = To Variant(anything=w1732) -> (Variant=w1731:variant)
        n312 = To Variant(anything=w1728) -> (Variant=w1727:variant)
        n313 = To Variant(anything=w1730) -> (Variant=w1729:variant)
        n314 = And(x=w1753, y=w1754) -> (x .and. y?=w1752:bool)
        n315 = And(x=w1757, y=w1752) -> (x .and. y?=w1756:bool)
        n316 = Variant To Data(error in=w1758, Variant=w1703) -> (data=→"Test Interval (Sec)":i32, error out=w1749:errorcluster)  [unwired: 1 in]
        n317 = Variant To Data(error in=w1755, Variant=w1701) -> (data=→"Test Interval Fault":bool, error out=w1748:errorcluster)  [unwired: 1 in]
        n318 = And(x=w1776, y=w1756) -> (x .and. y?=w1775:bool)
        n319 = And(x=w1790, y=w1775) -> (x .and. y?=w1791:bool)
        n320 = And(x=w1794, y=w1791) -> (x .and. y?=w1793:bool)
        n321 = And(x=w1798, y=w1793) -> (x .and. y?=w1797:bool)
        n322 = And(x=w1803, y=w1797) -> (x .and. y?=w1802:bool)
        n323 = And(x=w1816, y=w1802) -> (x .and. y?=w1817:bool)
        n324 = And(x=w1818, y=w1817) -> (x .and. y?=w1819:bool)
        n325 = And(x=w1821, y=w1819) -> (x .and. y?=w1820:bool)
        n326 = And(x=w1823, y=w1820) -> (x .and. y?=w1822:bool)
        n327 = And(x=w1908, y=w1822) -> (x .and. y?=w1924:bool)
        n328 = And(x=w1923, y=w1924) -> (x .and. y?=w1922:bool)
        n329 = And(x=w1921, y=w1922) -> (x .and. y?=w1920:bool)
        n330 = And(x=w1919, y=w1920) -> (x .and. y?=w1918:bool)
        n331 = And(x=w1917, y=w1918) -> (x .and. y?=w1916:bool)
        n332 = And(x=w1915, y=w1916) -> (x .and. y?=w1914:bool)
        n333 = And(x=w1925, y=w1914) -> (x .and. y?=w1877:bool)
        n334 = And(x=w1876, y=w1877) -> (x .and. y?=w1875:bool)
        n335 = And(x=w1874, y=w1875) -> (x .and. y?=w1873:bool)
        n336 = And(x=w1872, y=w1873) -> (x .and. y?=w1825:bool)
        n337 = And(x=w1826, y=w1825) -> (x .and. y?=w1824:bool)
        n338 = And(x=w1884, y=w1824) -> (x .and. y?=w1883:bool)
        n339 = And(x=w1885, y=w1883) -> (x .and. y?=w1882:bool)
        n340 = And(x=w1891, y=w1882) -> (x .and. y?=w1890:bool)
        n341 = And(x=w1929, y=w1890) -> (x .and. y?=w1928:bool)
        n342 = Variant To Data(error in=w1834, Variant=w1745) -> (data=→"Cap 1 Voltage (HVPS)":i16, error out=w1832:errorcluster)  [unwired: 1 in]
        n343 = Variant To Data(error in=w1907, Variant=w1735) -> (data=→"Discharge Fault":bool, error out=w1854:errorcluster)  [unwired: 1 in]
        n344 = Variant To Data(error in=w1926, Variant=w1737) -> (data=→"Charge Fault":bool, error out=w1852:errorcluster)  [unwired: 1 in]
        n345 = Variant To Data(error in=w1905, Variant=w1731) -> (data=→"Cap 1 Temp\nExceeded Fault":bool, error out=w1858:errorcluster)  [unwired: 1 in]
        n346 = And(x=w1927, y=w1928) -> (x .and. y?=→"Read Status":bool)
        n347 = Variant To Data(error in=w1906, Variant=w1733) -> (data=→"Hold Fault":bool, error out=w1856:errorcluster)  [unwired: 1 in]
        n348 = Variant To Data(error in=w1871, Variant=w1743) -> (data=→"Load Temperature":i16, error out=w1837:errorcluster)  [unwired: 1 in]
        n349 = Variant To Data(error in=w1904, Variant=w1729) -> (data=→"Ambient Temp\nExceeded Fault":bool, error out=w1860:errorcluster)  [unwired: 1 in]
        n350 = Variant To Data(error in=w1903, Variant=w1727) -> (data=→"PSU Fault":bool, error out=w1862:errorcluster)  [unwired: 1 in]
        n351 = Variant To Data(error in=w1902, Variant=w1725) -> (data=→"Control Sys Fault":bool, error out=w1864:errorcluster)  [unwired: 1 in]
        n352 = Variant To Data(error in=w1893, Variant=w1723) -> (data=→"test Running":bool, error out=w1865:errorcluster)  [unwired: 1 in]
        n353 = Variant To Data(error in=w1869, Variant=w1739) -> (data=→"Ambient Temp":i16, error out=w1850:errorcluster)  [unwired: 1 in]
        n354 = Variant To Data(error in=w1810, Variant=w1715) -> (data=w1805:bool, error out=w1808:errorcluster)  [unwired: 1 in]
        "Soft Exception" <- w1805
        n355 = Variant To Data(error in=w1801, Variant=w1713) -> (data=w1799:bool, error out=w1782:errorcluster)  [unwired: 1 in]
        "EOC" <- w1799
        n356 = Variant To Data(error in=w1870, Variant=w1741) -> (data=→"Soft Dump Temp":i16, error out=w1848:errorcluster)  [unwired: 1 in]
        n357 = Variant To Data(error in=w1815, Variant=w1721) -> (data=w1800:bool, error out=w1814:errorcluster)  [unwired: 1 in]
        "Softdump FB Fault" <- w1800
        n358 = Variant To Data(error in=w1811, Variant=w1717) -> (data=w1806:bool, error out=w1809:errorcluster)  [unwired: 1 in]
        "PSU HV FB Fault" <- w1806
        n359 = Variant To Data(error in=w1796, Variant=w1711) -> (data=w1770:bool, error out=w1781:errorcluster)  [unwired: 1 in]
        "SCR Ready" <- w1770
        n360 = Variant To Data(error in=w1795, Variant=w1709) -> (data=→"Maximum Test Number Reached":bool, error out=w1780:errorcluster)  [unwired: 1 in]
        n361 = Variant To Data(error in=w1813, Variant=w1719) -> (data=w1807:bool, error out=w1812:errorcluster)  [unwired: 1 in]
        "Charge FB Fault" <- w1807
        n362 = Variant To Data(error in=w1774, Variant=w1705) -> (data=w1771:bool, error out=w1773:errorcluster)  [unwired: 1 in]
        "Scope Trig" <- w1771
        n363 = Variant To Data(error in=w1888, type=2, Variant=w1889) -> (data=w1772:i32, error out=w1843:errorcluster)
        "Process Step" <- w1772
        n364 = Variant To Data(error in=w1881, Variant=w1878) -> (data=→"Cap 1 Temperature":i16, error out=w1847:errorcluster)  [unwired: 1 in]
        n365 = Variant To Data(error in=w1880, Variant=w1879) -> (data=w1788:i16, error out=w1845:errorcluster)  [unwired: 1 in]
        "Cap 1 Voltage" <- w1788
        n366 = Variant To Data(error in=w1789, Variant=w1707) -> (data=w1778:i16, error out=w1779:errorcluster)  [unwired: 1 in]
        "Expected Voltage" <- w1778
        n367 = Variant To Data(error in=w1913, Variant=w1912) -> (data=→"Estimated Charge Time (seconds)":sgl, error out=w1839:errorcluster)  [unwired: 1 in]
        n368 = To Double Precision Float(number=w1788) -> (double precision float=→"Waveform Chart - Capacitor Voltage (Probe, abs(Volts))":dbl)
        n369 = Variant To Data(error in=w1892, Variant=w1911) -> (data=→"Shot Number":i16, error out=w1841:errorcluster)  [unwired: 1 in]
        n370 = case shown="True" "Log Temperature Data" {
          tunnel: [errorcluster {"status"=FALSE, "code"=0, "source"=""} ("error out") w1939] -> w1831
          frame False {
          }
          frame True {
            n371 = local read "Cap 1 Temperature"() -> (w1940:i16)
            n372 = local read "test Running"() -> (w1938:bool)
            n373 = call "Write To Measurement File2"("Signals"=w1940, "Enable"=w1938, "Filename"="Capacitor Temperature Data Log File Path (.xlsx)") -> ("error out"=w1939:errorcluster)  [unwired: 14 in, 2 out]
          }
        }
        n374 = case shown="2" w1772 {
          tunnel: ["Charge" "Current Controlled Charge" "Hold - Ready for Shot" "Hold - Cap Open Circuited" "Shot" "Wait" "Dump" "Error" "Wait"] -> w1887
          tunnel: [TRUE TRUE TRUE TRUE TRUE TRUE FALSE FALSE FALSE] -> w1768
          tunnel: [FALSE ("Reset") FALSE ("Reset") FALSE ("Reset") FALSE ("Reset") TRUE ("Reset") FALSE ("Reset") FALSE ("Reset") TRUE ("Reset") FALSE ("Reset")] -> _
          frame 1 {
          }
          frame 6 {
          }
          frame 2 {
          }
          frame 7 {
          }
          frame 3 {
          }
          frame 4 {
          }
          frame 5 {
          }
          frame 99 {
          }
          frame 0, Default {
          }
        }
        "Test State" <- w1887
        n375 = local write "Scope Trig"(w1771) -> ()
        n376 = local read "Cap 1 Voltage"() -> (w1760:i16)
        n377 = case shown="True" "Log Capacitor Voltage" {
          tunnel: [errorcluster {"status"=FALSE, "code"=0, "source"=""} ("error out") w1936] -> w1829
          tunnel: w1788 -> [_ w1935]
          tunnel: w1768 -> [_ w1934]
          frame False {
          }
          frame True {
            n378 = local read "test Running"() -> (w1931:bool)
            n379 = And(x=w1934, y=w1931) -> (x .and. y?=w1932:bool)
            n380 = call "Write To Measurement File"("Signals"=w1935, "Enable"=w1932, "Filename"="Capacitor Voltage Data Log File Path (.xlsx)") -> ("error out"=w1936:errorcluster)  [unwired: 14 in, 2 out]
          }
        }
        n381 = Not(x=w1799) -> (.not. x?=w1786:bool)
        n382 = To Double Precision Float(number=w1760) -> (double precision float=w1784:dbl)
        n383 = To Double Precision Float(number=w1778) -> (double precision float=w1777:dbl)
        n384 = Boolean To (0,1)(Boolean=w1786) -> (0, 1=→"EOC":i16)
        n385 = Or(x=w1864, y=w1865) -> (x .or. y?=w1863:bool)
        n386 = Or(x=w1862, y=w1863) -> (x .or. y?=w1861:bool)
        n387 = Or(x=w1860, y=w1861) -> (x .or. y?=w1859:bool)
        n388 = Or(x=w1858, y=w1859) -> (x .or. y?=w1857:bool)
        n389 = Or(x=w1856, y=w1857) -> (x .or. y?=w1855:bool)
        n390 = Or(x=w1854, y=w1855) -> (x .or. y?=w1853:bool)
        n391 = Or(x=w1852, y=w1853) -> (x .or. y?=w1851:bool)
        n392 = Or(x=w1850, y=w1851) -> (x .or. y?=w1849:bool)
        n393 = Or(x=w1848, y=w1849) -> (x .or. y?=w1836:bool)
        n394 = Or(x=w1837, y=w1836) -> (x .or. y?=w1830:bool)
        n395 = Boolean To (0,1)(Boolean=w1770) -> (0, 1=→"SCR FB":i16)
        n396 = Bundle(w1784, w1777) -> (→"Capacitor Voltage":cluster{dbl, dbl})  [unwired: 1 in]
        n397 = local write "Process Step"(w1772) -> ()
        n398 = local read "Scope Trig"() -> (w1763:bool)
        n399 = local read "Test Interval (Sec)"() -> (w1766:i32)
        n400 = Not(x=w1763) -> (.not. x?=w1762:bool)
        n401 = call "Elapsed Time"("Time Target (s)"=w1766, "Reset"=w1762) -> ("Elapsed Time Text"=w1765:string)  [unwired: 10 in, 7 out]
        n402 = String Subset(string=w1765, offset (0)=2) -> (substring=→"Time Since Last Shot":string)  [unwired: 1 in]
        n403 = Or(x=w1831, y=w1830) -> (x .or. y?=w1828:bool)
        n404 = Or(x=w1829, y=w1828) -> (x .or. y?=w1827:bool)
        n405 = Or(x=w1847, y=w1827) -> (x .or. y?=w1846:bool)
        n406 = Or(x=w1845, y=w1846) -> (x .or. y?=w1844:bool)
        n407 = Or(x=w1843, y=w1844) -> (x .or. y?=w1842:bool)
        n408 = Or(x=w1841, y=w1842) -> (x .or. y?=w1840:bool)
        n409 = Or(x=w1839, y=w1840) -> (x .or. y?=w1838:bool)
        "Internal TwinCAT Handle ID Maps" <- w1747
      }
    }
    n410 = call-poly <userlib>:"Write TypeResolved.vi"("Handle"=w518, "SymbolName"=w539, "WData"=w535, "error constant"=w514) -> ("Write Status?"=w506:bool, "Has Matched?"=w509:bool, "error out"=w533:errorcluster)  [unwired: 8 in, 1 out]
    n411 = call-poly <userlib>:"Write TypeResolved.vi"("Handle"=w518, "SymbolName"=w540, "WData"=w536, "error constant"=w514) -> ("Write Status?"=w505:bool, "Has Matched?"=w510:bool, "error out"=w534:errorcluster)  [unwired: 8 in, 1 out]
    n412 = call <userlib>:"Send Writer-Request.vi"("Handle"=w1055, "SymbolName"=w1054, "WriterMode"=w1053, "WriteHandle"=w1052, "error constant"=w1051, "ADS Write Data"=w779) -> ("Handle"=w1047:u32, "WriteHandle"=w1046:u32, "Write status?"=w757:bool, "error IO"=w711:errorcluster)  [unwired: 5 in, 1 out]
    n413 = call-poly <userlib>:"Write TypeResolved.vi"("Handle"=w518, "SymbolName"=w556, "WData"=w548, "error constant"=w555) -> ("Handle"=w549:u32, "Write Status?"=w504:bool, "Has Matched?"=w512:bool, "error out"=w550:errorcluster)  [unwired: 8 in]
    n414 = call <userlib>:"Send Writer-Request.vi"("Handle"=w489, "SymbolName"=w490, "WriterMode"=w802, "WriteHandle"=w800, "error constant"=w801, "ADS Write Data"=w491) -> ("Handle"=w796:u32, "WriteHandle"=w795:u32, "Write status?"=w628:bool, "error IO"=w486:errorcluster)  [unwired: 5 in, 1 out]
    n415 = call <userlib>:"Send Writer-Request.vi"("Handle"=w644, "SymbolName"=w643, "WriterMode"=w642, "WriteHandle"=w641, "error constant"=w640, "ADS Write Data"=w636) -> ("Handle"=w635:u32, "WriteHandle"=w632:u32, "Write status?"=w554:bool, "error IO"=w484:errorcluster)  [unwired: 5 in, 1 out]
    n416 = call <userlib>:"Send Writer-Request.vi"("Handle"=w971, "SymbolName"=w970, "WriterMode"=w969, "WriteHandle"=w967, "error constant"=w968, "ADS Write Data"=w878) -> ("Handle"=w966:u32, "WriteHandle"=w965:u32, "Write status?"=w530:bool, "error IO"=w691:errorcluster)  [unwired: 5 in, 1 out]
    n417 = call <userlib>:"Send Writer-Request.vi"("Handle"=w911, "SymbolName"=w910, "WriterMode"=w909, "WriteHandle"=w908, "error constant"=w907, "ADS Write Data"=w873) -> ("Handle"=w903:u32, "WriteHandle"=w902:u32, "Write status?"=w525:bool, "error IO"=w676:errorcluster)  [unwired: 5 in, 1 out]
    n418 = call <userlib>:"Send Writer-Request.vi"("Handle"=w868, "SymbolName"=w867, "WriterMode"=w866, "WriteHandle"=w857, "error constant"=w865, "ADS Write Data"=w492) -> ("Handle"=w864:u32, "WriteHandle"=w863:u32, "Write status?"=w524:bool, "error IO"=w488:errorcluster)  [unwired: 5 in, 1 out]
    n419 = call <userlib>:"Send Writer-Request.vi"("Handle"=w959, "SymbolName"=w958, "WriterMode"=w957, "WriteHandle"=w956, "error constant"=w955, "ADS Write Data"=w877) -> ("Handle"=w951:u32, "WriteHandle"=w950:u32, "Write status?"=w529:bool, "error IO"=w688:errorcluster)  [unwired: 5 in, 1 out]
    n420 = call <userlib>:"Send Writer-Request.vi"("Handle"=w935, "SymbolName"=w934, "WriterMode"=w933, "WriteHandle"=w932, "error constant"=w931, "ADS Write Data"=w875) -> ("Handle"=w927:u32, "WriteHandle"=w926:u32, "Write status?"=w527:bool, "error IO"=w682:errorcluster)  [unwired: 5 in, 1 out]
    n421 = call <userlib>:"Send Writer-Request.vi"("Handle"=w947, "SymbolName"=w946, "WriterMode"=w945, "WriteHandle"=w944, "error constant"=w943, "ADS Write Data"=w876) -> ("Handle"=w939:u32, "WriteHandle"=w938:u32, "Write status?"=w528:bool, "error IO"=w685:errorcluster)  [unwired: 5 in, 1 out]
    n422 = call <userlib>:"Send Writer-Request.vi"("Handle"=w923, "SymbolName"=w922, "WriterMode"=w921, "WriteHandle"=w920, "error constant"=w919, "ADS Write Data"=w874) -> ("Handle"=w915:u32, "WriteHandle"=w914:u32, "Write status?"=w526:bool, "error IO"=w679:errorcluster)  [unwired: 5 in, 1 out]
    n423 = call <userlib>:"Send Writer-Request.vi"("Handle"=w1043, "SymbolName"=w1042, "WriterMode"=w1041, "WriteHandle"=w1039, "error constant"=w1040, "ADS Write Data"=w884) -> ("Handle"=w1038:u32, "WriteHandle"=w1037:u32, "Write status?"=w745:bool, "error IO"=w708:errorcluster)  [unwired: 5 in, 1 out]
    n424 = call <userlib>:"Send Writer-Request.vi"("Handle"=w983, "SymbolName"=w982, "WriterMode"=w981, "WriteHandle"=w980, "error constant"=w979, "ADS Write Data"=w879) -> ("Handle"=w975:u32, "WriteHandle"=w974:u32, "Write status?"=w755:bool, "error IO"=w693:errorcluster)  [unwired: 5 in, 1 out]
    n425 = call <userlib>:"Send Writer-Request.vi"("Handle"=w1031, "SymbolName"=w1030, "WriterMode"=w1029, "WriteHandle"=w1028, "error constant"=w1027, "ADS Write Data"=w883) -> ("Handle"=w1023:u32, "WriteHandle"=w1022:u32, "Write status?"=w747:bool, "error IO"=w705:errorcluster)  [unwired: 5 in, 1 out]
    n426 = call <userlib>:"Send Writer-Request.vi"("Handle"=w1007, "SymbolName"=w1006, "WriterMode"=w1005, "WriteHandle"=w1004, "error constant"=w1003, "ADS Write Data"=w881) -> ("Handle"=w999:u32, "WriteHandle"=w998:u32, "Write status?"=w751:bool, "error IO"=w699:errorcluster)  [unwired: 5 in, 1 out]
    n427 = call <userlib>:"Send Writer-Request.vi"("Handle"=w1019, "SymbolName"=w1018, "WriterMode"=w1017, "WriteHandle"=w1016, "error constant"=w1015, "ADS Write Data"=w882) -> ("Handle"=w1011:u32, "WriteHandle"=w1010:u32, "Write status?"=w749:bool, "error IO"=w702:errorcluster)  [unwired: 5 in, 1 out]
    n428 = call <userlib>:"Send Writer-Request.vi"("Handle"=w995, "SymbolName"=w994, "WriterMode"=w993, "WriteHandle"=w992, "error constant"=w991, "ADS Write Data"=w880) -> ("Handle"=w987:u32, "WriteHandle"=w986:u32, "Write status?"=w753:bool, "error IO"=w696:errorcluster)  [unwired: 5 in, 1 out]
    n429 = call <userlib>:"Send Writer-Request.vi"("Handle"=w666, "SymbolName"=w665, "WriterMode"=w664, "WriteHandle"=w663, "error constant"=w662, "ADS Write Data"=w658) -> ("Handle"=w657:u32, "WriteHandle"=w656:u32, "Write status?"=w650:bool, "error IO"=w481:errorcluster)  [unwired: 5 in, 1 out]
    n430 = Compound Arithmetic op=AND(w512, w510, w509, w508) -> (w511:bool)
    n431 = And(x=w552, y=w511) -> (x .and. y?=w551:bool)
    n432 = And(x=w631, y=w551) -> (x .and. y?=w630:bool)
    n433 = And(x=w741, y=w630) -> (x .and. y?=w740:bool)
    n434 = And(x=w739, y=w740) -> (x .and. y?=w738:bool)
    n435 = And(x=w737, y=w738) -> (x .and. y?=w736:bool)
    n436 = And(x=w735, y=w736) -> (x .and. y?=w734:bool)
    n437 = And(x=w733, y=w734) -> (x .and. y?=w732:bool)
    n438 = And(x=w731, y=w732) -> (x .and. y?=w730:bool)
    n439 = And(x=w729, y=w730) -> (x .and. y?=w621:bool)
    n440 = And(x=w652, y=w621) -> (x .and. y?=w653:bool)
    n441 = And(x=w728, y=w653) -> (x .and. y?=w727:bool)
    n442 = And(x=w726, y=w727) -> (x .and. y?=w725:bool)
    n443 = And(x=w724, y=w725) -> (x .and. y?=w723:bool)
    n444 = And(x=w722, y=w723) -> (x .and. y?=w721:bool)
    n445 = And(x=w720, y=w721) -> (x .and. y?=w719:bool)
    n446 = And(x=w718, y=w719) -> (x .and. y?=w717:bool)
    n447 = And(x=w716, y=w717) -> (x .and. y?=w715:bool)
    n448 = And(x=w743, y=w715) -> (x .and. y?=→"bHasMached":bool)
    n449 = Compound Arithmetic op=AND(w504, w505, w506, w507) -> (w503:bool)
    n450 = And(x=w554, y=w503) -> (x .and. y?=w553:bool)
    n451 = And(x=w628, y=w553) -> (x .and. y?=w521:bool)
    n452 = Compound Arithmetic op=AND(w530, w529, w528, w527, w526, w525, w524) -> (w523:bool)
    n453 = Not(x=w523) -> (.not. x?=w522:bool)
    n454 = And(x=w522, y=w521) -> (x .and. y?=w520:bool)
    n455 = And(x=w650, y=w520) -> (x .and. y?=w651:bool)
    n456 = And(x=w755, y=w651) -> (x .and. y?=w754:bool)
    n457 = And(x=w753, y=w754) -> (x .and. y?=w752:bool)
    n458 = And(x=w751, y=w752) -> (x .and. y?=w750:bool)
    n459 = And(x=w749, y=w750) -> (x .and. y?=w748:bool)
    n460 = And(x=w747, y=w748) -> (x .and. y?=w746:bool)
    n461 = And(x=w745, y=w746) -> (x .and. y?=w744:bool)
    n462 = And(x=w757, y=w744) -> (x .and. y?=w756:bool)
    n463 = And(x=w758, y=w756) -> (x .and. y?=→"Write Status":bool)
    n464 = feedback #2(TRUE) -> (w576:bool)
    n465 = And(x=w576, y=w579) -> (x .and. y?=w578:bool)
    n466 = feedback #3(TRUE) -> (w586:bool)
    n467 = And(x=w586, y=w589) -> (x .and. y?=w588:bool)
    n468 = Compound Arithmetic op=OR("EXIT HMI") -> (w618:bool)
    "Stop Loops" <- w618
    n469 = feedback #4(TRUE) -> (w590:bool)
    n470 = And(x=w590, y=w593) -> (x .and. y?=w592:bool)
    n471 = feedback #5(TRUE) -> (w582:bool)
    n472 = And(x=w582, y=w581) -> (x .and. y?=w583:bool)
    n473 = case shown="True" w583 {
      tunnel: [w1254 FALSE] -> w573
      tunnel: w574 -> [w1256 _]
      frame False {
        n474 = Or(x=w1256, y=FALSE) -> (x .or. y?=w1254:bool)
      }
      frame True {
        n475 = call "Charge relay error"() -> ()  [unwired: 10 in, 2 out]
      }
    }
    n476 = feedback-in #5(w573) -> ()
    n477 = case shown="True" w578 {
      tunnel: [w1252 FALSE] -> w577
      tunnel: w573 -> [w1250 _]
      frame False {
        n478 = Or(x=w1250, y=FALSE) -> (x .or. y?=w1252:bool)
      }
      frame True {
        n479 = call "PSU HV error"() -> ()  [unwired: 10 in, 2 out]
      }
    }
    n480 = feedback-in #2(w577) -> ()
    n481 = case shown="True" w592 {
      tunnel: [w1263 FALSE] -> w591
      tunnel: w574 -> [w1262 _]
      frame False {
        n482 = Or(x=w1262, y=FALSE) -> (x .or. y?=w1263:bool)
      }
      frame True {
        n483 = call "Softdump error"() -> ()  [unwired: 10 in, 2 out]
      }
    }
    n484 = feedback-in #4(w591) -> ()
    n485 = case shown="True" w588 {
      tunnel: [w1258 FALSE] -> w587
      tunnel: w573 -> [w1259 _]
      frame False {
        n486 = Or(x=w1259, y=FALSE) -> (x .or. y?=w1258:bool)
      }
      frame True {
        n487 = call "Soft Exception"() -> ()  [unwired: 10 in, 2 out]
      }
    }
    n488 = feedback-in #3(w587) -> ()
    n489 = Compound Arithmetic op=OR(w672, w714, w713) -> (w712:bool)
    n490 = Compound Arithmetic op=OR(w712, w711, w710) -> (w709:bool)
    n491 = property on="Stop Loops" class="Bool (strict)"("Val(Sgnl)"=w618) -> ()  [unwired: 2 in, 2 out]
    n492 = Compound Arithmetic op=OR(w709, w708, w707) -> (w706:bool)
    n493 = Compound Arithmetic op=OR(w706, w705, w704) -> (w703:bool)
    n494 = Compound Arithmetic op=OR(w703, w702, w701) -> (w700:bool)
    n495 = Compound Arithmetic op=OR(w700, w699, w698) -> (w697:bool)
    n496 = Compound Arithmetic op=OR(w697, w696, w695) -> (w694:bool)
    n497 = Compound Arithmetic op=OR(w694, w693, w692) -> (w649:bool)
    n498 = Compound Arithmetic op=OR(w649, w481, w480) -> (w620:bool)
    n499 = Compound Arithmetic op=OR(w620, w691, w690) -> (w689:bool)
    n500 = Compound Arithmetic op=OR(w689, w688, w687) -> (w686:bool)
    n501 = Compound Arithmetic op=OR(w686, w685, w684) -> (w683:bool)
    n502 = Compound Arithmetic op=OR(w683, w682, w681) -> (w680:bool)
    n503 = Compound Arithmetic op=OR(w680, w679, w678) -> (w677:bool)
    n504 = Compound Arithmetic op=OR(w677, w676, w675) -> (w674:bool)
    n505 = Compound Arithmetic op=OR(w674, w488, w487) -> (w673:bool)
    n506 = Compound Arithmetic op=OR(w673, w486, w485) -> (w629:bool)
    n507 = Compound Arithmetic op=OR(w629, w484, w483) -> ()  [unwired: 1 out]
    n508 = node-c288() -> ()  [unwired: 1 in, 1 out]
  }
  n509 = node-c288(w112) -> (w111:errorcluster)
  n510 = call <userlib>:"Release Writer.vi"("Handle"=w218, "WriteHandle"=w217, "error in (no error)"=w216) -> ("error out"=w212:errorcluster)  [unwired: 11 in, 1 out]
  n511 = call <userlib>:"Release Writer.vi"("Handle"=w314, "WriteHandle"=w313, "error in (no error)"=w312) -> ("error out"=w320:errorcluster)  [unwired: 11 in, 1 out]
  n512 = call <userlib>:"Release Writer.vi"("Handle"=w294, "WriteHandle"=w293, "error in (no error)"=w292) -> ("error out"=w288:errorcluster)  [unwired: 11 in, 1 out]
  n513 = call <userlib>:"Release Writer.vi"("Handle"=w256, "WriteHandle"=w255, "error in (no error)"=w254) -> ("error out"=w250:errorcluster)  [unwired: 11 in, 1 out]
  n514 = call <userlib>:"Release Type.vi"("Handle"=w215, "TypeHandle"=w214, "error in (no error)"=w213) -> ("error out"=w211:errorcluster)  [unwired: 11 in, 1 out]
  n515 = call <userlib>:"Release Type.vi"("Handle"=w309, "TypeHandle"=w310, "error in (no error)"=w311) -> ("error out"=w321:errorcluster)  [unwired: 11 in, 1 out]
  n516 = call <userlib>:"Release Type.vi"("Handle"=w291, "TypeHandle"=w290, "error in (no error)"=w289) -> ("error out"=w287:errorcluster)  [unwired: 11 in, 1 out]
  n517 = call <userlib>:"Release Writer.vi"("Handle"=w275, "WriteHandle"=w274, "error in (no error)"=w273) -> ("error out"=w269:errorcluster)  [unwired: 11 in, 1 out]
  n518 = call <userlib>:"Release Type.vi"("Handle"=w253, "TypeHandle"=w252, "error in (no error)"=w251) -> ("error out"=w249:errorcluster)  [unwired: 11 in, 1 out]
  n519 = call <userlib>:"Release Writer.vi"("Handle"=w237, "WriteHandle"=w236, "error in (no error)"=w235) -> ("error out"=w231:errorcluster)  [unwired: 11 in, 1 out]
  n520 = call <userlib>:"Release Type.vi"("Handle"=w272, "TypeHandle"=w271, "error in (no error)"=w270) -> ("error out"=w268:errorcluster)  [unwired: 11 in, 1 out]
  n521 = call <userlib>:"Release Type.vi"("Handle"=w234, "TypeHandle"=w233, "error in (no error)"=w232) -> ("error out"=w230:errorcluster)  [unwired: 11 in, 1 out]
  n522 = call <userlib>:"Release Type.vi"("Handle"=w7, "TypeHandle"=w8, "error in (no error)"=w6) -> ("error out"=w5:errorcluster)  [unwired: 11 in, 1 out]
  n523 = call <userlib>:"Release Writer.vi"("Handle"=w463, "WriteHandle"=w462, "error in (no error)"=w473) -> ("error out"=w145:errorcluster)  [unwired: 11 in, 1 out]
  n524 = call <userlib>:"Release Writer.vi"("Handle"=w332, "WriteHandle"=w331, "error in (no error)"=w330) -> ("error out"=w326:errorcluster)  [unwired: 11 in, 1 out]
  n525 = call <userlib>:"Release Writer.vi"("Handle"=w428, "WriteHandle"=w427, "error in (no error)"=w426) -> ("error out"=w434:errorcluster)  [unwired: 11 in, 1 out]
  n526 = call <userlib>:"Release Writer.vi"("Handle"=w408, "WriteHandle"=w407, "error in (no error)"=w406) -> ("error out"=w402:errorcluster)  [unwired: 11 in, 1 out]
  n527 = call <userlib>:"Release Writer.vi"("Handle"=w370, "WriteHandle"=w369, "error in (no error)"=w368) -> ("error out"=w364:errorcluster)  [unwired: 11 in, 1 out]
  n528 = call <userlib>:"Release Type.vi"("Handle"=w329, "TypeHandle"=w328, "error in (no error)"=w327) -> ("error out"=w325:errorcluster)  [unwired: 11 in, 1 out]
  n529 = call <userlib>:"Release Type.vi"("Handle"=w423, "TypeHandle"=w424, "error in (no error)"=w425) -> ("error out"=w435:errorcluster)  [unwired: 11 in, 1 out]
  n530 = call <userlib>:"Release Type.vi"("Handle"=w405, "TypeHandle"=w404, "error in (no error)"=w403) -> ("error out"=w401:errorcluster)  [unwired: 11 in, 1 out]
  n531 = call <userlib>:"Release Writer.vi"("Handle"=w389, "WriteHandle"=w388, "error in (no error)"=w387) -> ("error out"=w383:errorcluster)  [unwired: 11 in, 1 out]
  n532 = call <userlib>:"Release Type.vi"("Handle"=w367, "TypeHandle"=w366, "error in (no error)"=w365) -> ("error out"=w363:errorcluster)  [unwired: 11 in, 1 out]
  n533 = call <userlib>:"Release Writer.vi"("Handle"=w351, "WriteHandle"=w350, "error in (no error)"=w349) -> ("error out"=w345:errorcluster)  [unwired: 11 in, 1 out]
  n534 = call <userlib>:"Release Type.vi"("Handle"=w386, "TypeHandle"=w385, "error in (no error)"=w384) -> ("error out"=w382:errorcluster)  [unwired: 11 in, 1 out]
  n535 = call <userlib>:"Release Type.vi"("Handle"=w348, "TypeHandle"=w347, "error in (no error)"=w346) -> ("error out"=w344:errorcluster)  [unwired: 11 in, 1 out]
  n536 = call <userlib>:"Release Writer.vi"("Handle"=w446, "WriteHandle"=w445, "error in (no error)"=w444) -> ("error out"=w440:errorcluster)  [unwired: 11 in, 1 out]
  n537 = call <userlib>:"Release Writer.vi"("Handle"=w95, "WriteHandle"=w94, "error in (no error)"=w2) -> ("error out"=w109:errorcluster)  [unwired: 11 in, 1 out]
  n538 = call <userlib>:"Release Writer.vi"("Handle"=w9, "WriteHandle"=w181, "error in (no error)"=w20) -> ("error out"=w187:errorcluster)  [unwired: 11 in, 1 out]
  n539 = call <userlib>:"Release Type.vi"("Handle"=w443, "TypeHandle"=w442, "error in (no error)"=w441) -> ("error out"=w439:errorcluster)  [unwired: 11 in, 1 out]
  n540 = call <userlib>:"Release Type.vi"("Handle"=w93, "TypeHandle"=w92, "error in (no error)"=w1) -> ("error out"=w108:errorcluster)  [unwired: 11 in, 1 out]
  n541 = call <userlib>:"Release Type.vi"("Handle"=w177, "TypeHandle"=w176, "error in (no error)"=w19) -> ("error out"=w186:errorcluster)  [unwired: 11 in, 1 out]
  n542 = call <userlib>:"Release Writer.vi"("Handle"=w116, "WriteHandle"=w115, "error in (no error)"=w18) -> ("error out"=w117:errorcluster)  [unwired: 11 in, 1 out]
  n543 = call <userlib>:"Release Writer.vi"("Handle"=w15, "WriteHandle"=w14, "error in (no error)"=w17) -> ("Handle"=w4:u32, "error out"=w89:errorcluster)  [unwired: 11 in]
  n544 = call <userlib>:"Release Type.vi"("Handle"=w12, "TypeHandle"=w13, "error in (no error)"=w16) -> ("error out"=w88:errorcluster)  [unwired: 11 in, 1 out]
  n545 = call <userlib>:"Release Type.vi"("Handle"=w461, "TypeHandle"=w460, "error in (no error)"=w472) -> ("error out"=w146:errorcluster)  [unwired: 11 in, 1 out]
  n546 = Merge Errors(w320, w321) -> (w134:errorcluster)
  n547 = Merge Errors(w212, w211) -> (w129:errorcluster)
  n548 = Merge Errors(w288, w287) -> (w133:errorcluster)
  n549 = Merge Errors(w250, w249) -> (w131:errorcluster)
  n550 = Merge Errors(w269, w268) -> (w132:errorcluster)
  n551 = Merge Errors(w231, w230) -> (w130:errorcluster)
  n552 = Merge Errors(w434, w435) -> (w140:errorcluster)
  n553 = Merge Errors(w326, w325) -> (w135:errorcluster)
  n554 = Merge Errors(w402, w401) -> (w139:errorcluster)
  n555 = Merge Errors(w364, w363) -> (w137:errorcluster)
  n556 = Merge Errors(w383, w382) -> (w138:errorcluster)
  n557 = Merge Errors(w345, w344) -> (w136:errorcluster)
  n558 = Merge Errors(w440, w439) -> (w141:errorcluster)
  n559 = Merge Errors(w109, w108) -> (w107:errorcluster)
  n560 = Merge Errors(w187, w186) -> (w128:errorcluster)
  n561 = Merge Errors(w117, w5) -> (w114:errorcluster)
  n562 = Merge Errors(w89, w88) -> (w79:errorcluster)
  n563 = Merge Errors(w145, w146) -> (w144:errorcluster)
  n564 = Merge Errors(w51, w50, w49, w48, w40, w22, w21) -> (w46:errorcluster)
  n565 = Merge Errors(w140, w139, w138, w137, w136, w135, w107) -> (w204:errorcluster)
  n566 = Merge Errors(w134, w133, w132, w131, w130, w129, w128, w114, w79, w35, w34, w33, w29) -> (w203:errorcluster)
  n567 = Merge Errors(w156, w157, w158, w159, w160, w76, w75, w71, w72, w73, w74) -> (w147:errorcluster)
  n568 = Merge Errors(w110, w155, w154, w153, w152, w151, w150, w149, w62, w61, w60, w47, w46) -> (w148:errorcluster)
  n569 = Merge Errors(w147, w148) -> (w28:errorcluster)
  n570 = Merge Errors(w111, w144, w141, w204, w203, w28) -> (w142:errorcluster)
  n571 = call <userlib>:"Release.vi"("Handle"=w4, "error in (no error)"=w142) -> ("error out"=→"error out":errorcluster)  [unwired: 13 in]
